vi "statistical test.vi"() -> ()   [LabVIEW 2020]
uses:
  cbe3630c-a9ac-4615-a769-21536e683349.vi
  c04601fd-c9b4-47d5-8825-3c995806f4c0.vi
  2572ad4a-3046-4405-892d-2e3ff8b2e1b5.vi
  <vilib>/Analysis/2dsp.llb/Real FFT.vi
  e90844b8-1ebf-47aa-9ece-e238ecb31719.vi
  c1b2c77b-ae4a-4a6f-8510-2936ba5ac98e.vi
  64edd431-45f5-4cf3-b232-8b968e9fa659.vi
  ced42c1c-8a2c-4fd2-8d95-4dc111501514.vi
  3b9e0fed-1065-4ad9-a1c5-79d92d83ef64.vi
  <vilib>/Utility/file.llb/Read Delimited Spreadsheet (string).vi
  <vilib>/gmath/statdist.llb/Normal CDF.vi
  <vilib>/Comparison/Equal/Equal Functor/Equal Functor.lvclass
  <vilib>/express/express arith-compare/Formula/XNode/ExpressFormulaBlockNode.xnode
  <vilib>/gmath/NI_Gmath.lvlib
  <vilib>/Analysis/NI_AALPro.lvlib
panel:
  out "size(s)":i32
  in  "?":T1(tab)
  out "?":dbl
  out "?":dbl format="%.6f"
  out "?":dbl format="%.6f"
  out "?":dbl format="%.6f"
  out "?":dbl
  out "1 - erf(x)":dbl format="%.6f"
  out "1 - g(x, a)":dbl format="%.6f"
  out "P-VALUE 2":dbl format="%.6f"
  out "p-value 4":dbl format="%.6f"
  out "?":dbl format="%.6f"
  out "?":dbl format="%.6f"
  out "?":dbl format="%.6f"
  out "?":dbl
  out "?":dbl
  out "?":dbl
  out "?":string
  out "?":string
  out "?":string
  out "?":string
  out "?":string
  out "?":string
  out "?":string
  out "?":string
  out "?":string
  out "?":string
  out "?":string
  out "?":string
  out "?":string
  out "?":string
  out "?":string
  out "lxl":i32
  out "Z-":i32
  out "s":dbl
  out "sqrt(Z-)":dbl
  out "s/sqrt(2)":dbl
  out "X":dbl format="%#_8g"
  out "X/2":dbl format="%#_8g"
  out "n/2":dbl
  in  "M 길이":i32
  out "pi":dbl
  out "V(obs)":i32
  out "erfc(  )":dbl
  in  "MAX RUN":i32
  out "X^2":dbl
  out "Array":i32[](array[numeric])
  out "N":dbl
  out "32":dbl
  out "31":dbl
  out "0":dbl
  out "X^2 2":dbl format="%#_8g"
  out "결과":dbl
  in  "차원 크기":i32
  out "log(x)":dbl
  out "T":dbl
  out "N0":dbl format="%#_8g"
  out "N1":dbl format="%#_8g"
  out "x":dbl
  out "d":dbl
  out "u":dbl
  out "시그마^2":dbl
  out "X^2 3":dbl
  out "길이 M":i32
  out "람다":dbl
  out "에타":dbl
  out "v4":i32
  out "v1":i32
  out "v0":i32
  out "v5":i32
  out "v2":i32
  out "v3":i32
  out "X^2 4":dbl format="%#_7g"
  out "f(n)":dbl
  out "c":dbl
  out "시그마":dbl
  out "erfc( )":dbl
  in  "dimension size":i32
  out "v0 2":i32
  out "v1 2":i32
  out "v2 2":i32
  out "v3 2":i32
  out "v4 2":i32
  out "v5 2":i32
  out "v6":i32
  out "전체":i32
  out "안에":i32
  in  "m":i32
  out "델타 프사이":dbl
  out "델타^2 프사이":dbl
  out "2^(m-2)":dbl
  out "2^(m-3)":dbl
  out "p-value2":dbl format="%.6f"
  in  "m 2":i32
  out "ApEn(m)":dbl
  out "X^2 5":dbl format="%#_7g"
  out "forward max value":i32
  out "backward max value":i32
  out "backward P-value":dbl
  out "Forward P-value":dbl
  out "J":i32
  out "P- VALUE":dbl[](array[numeric])
  out "X^2 6":dbl[](array[numeric])
  out "J":i32
  out "P-VALUE":dbl[](array[numeric])
  out "Numeric 3":i32 format="%b"
  out "Numeric 2":i32 format="%b"
  # "Statistical Test                 P-value              Result"
  # "Frequency"
  # "Block Frequency"
  # "Runs"
  # "Long Runs of Ones"
  # "Rank"
  # "FFT"
  # "NON-overlapping Templates"
  # "Overlapping Templates"
  # "Universal"
  # "Linear Complexity"
  # "Serial"
  # "Approximate Entropy"
  # "Cumulative  sum"
  # "Random Excursious"
  # "Random Excursious Variant"
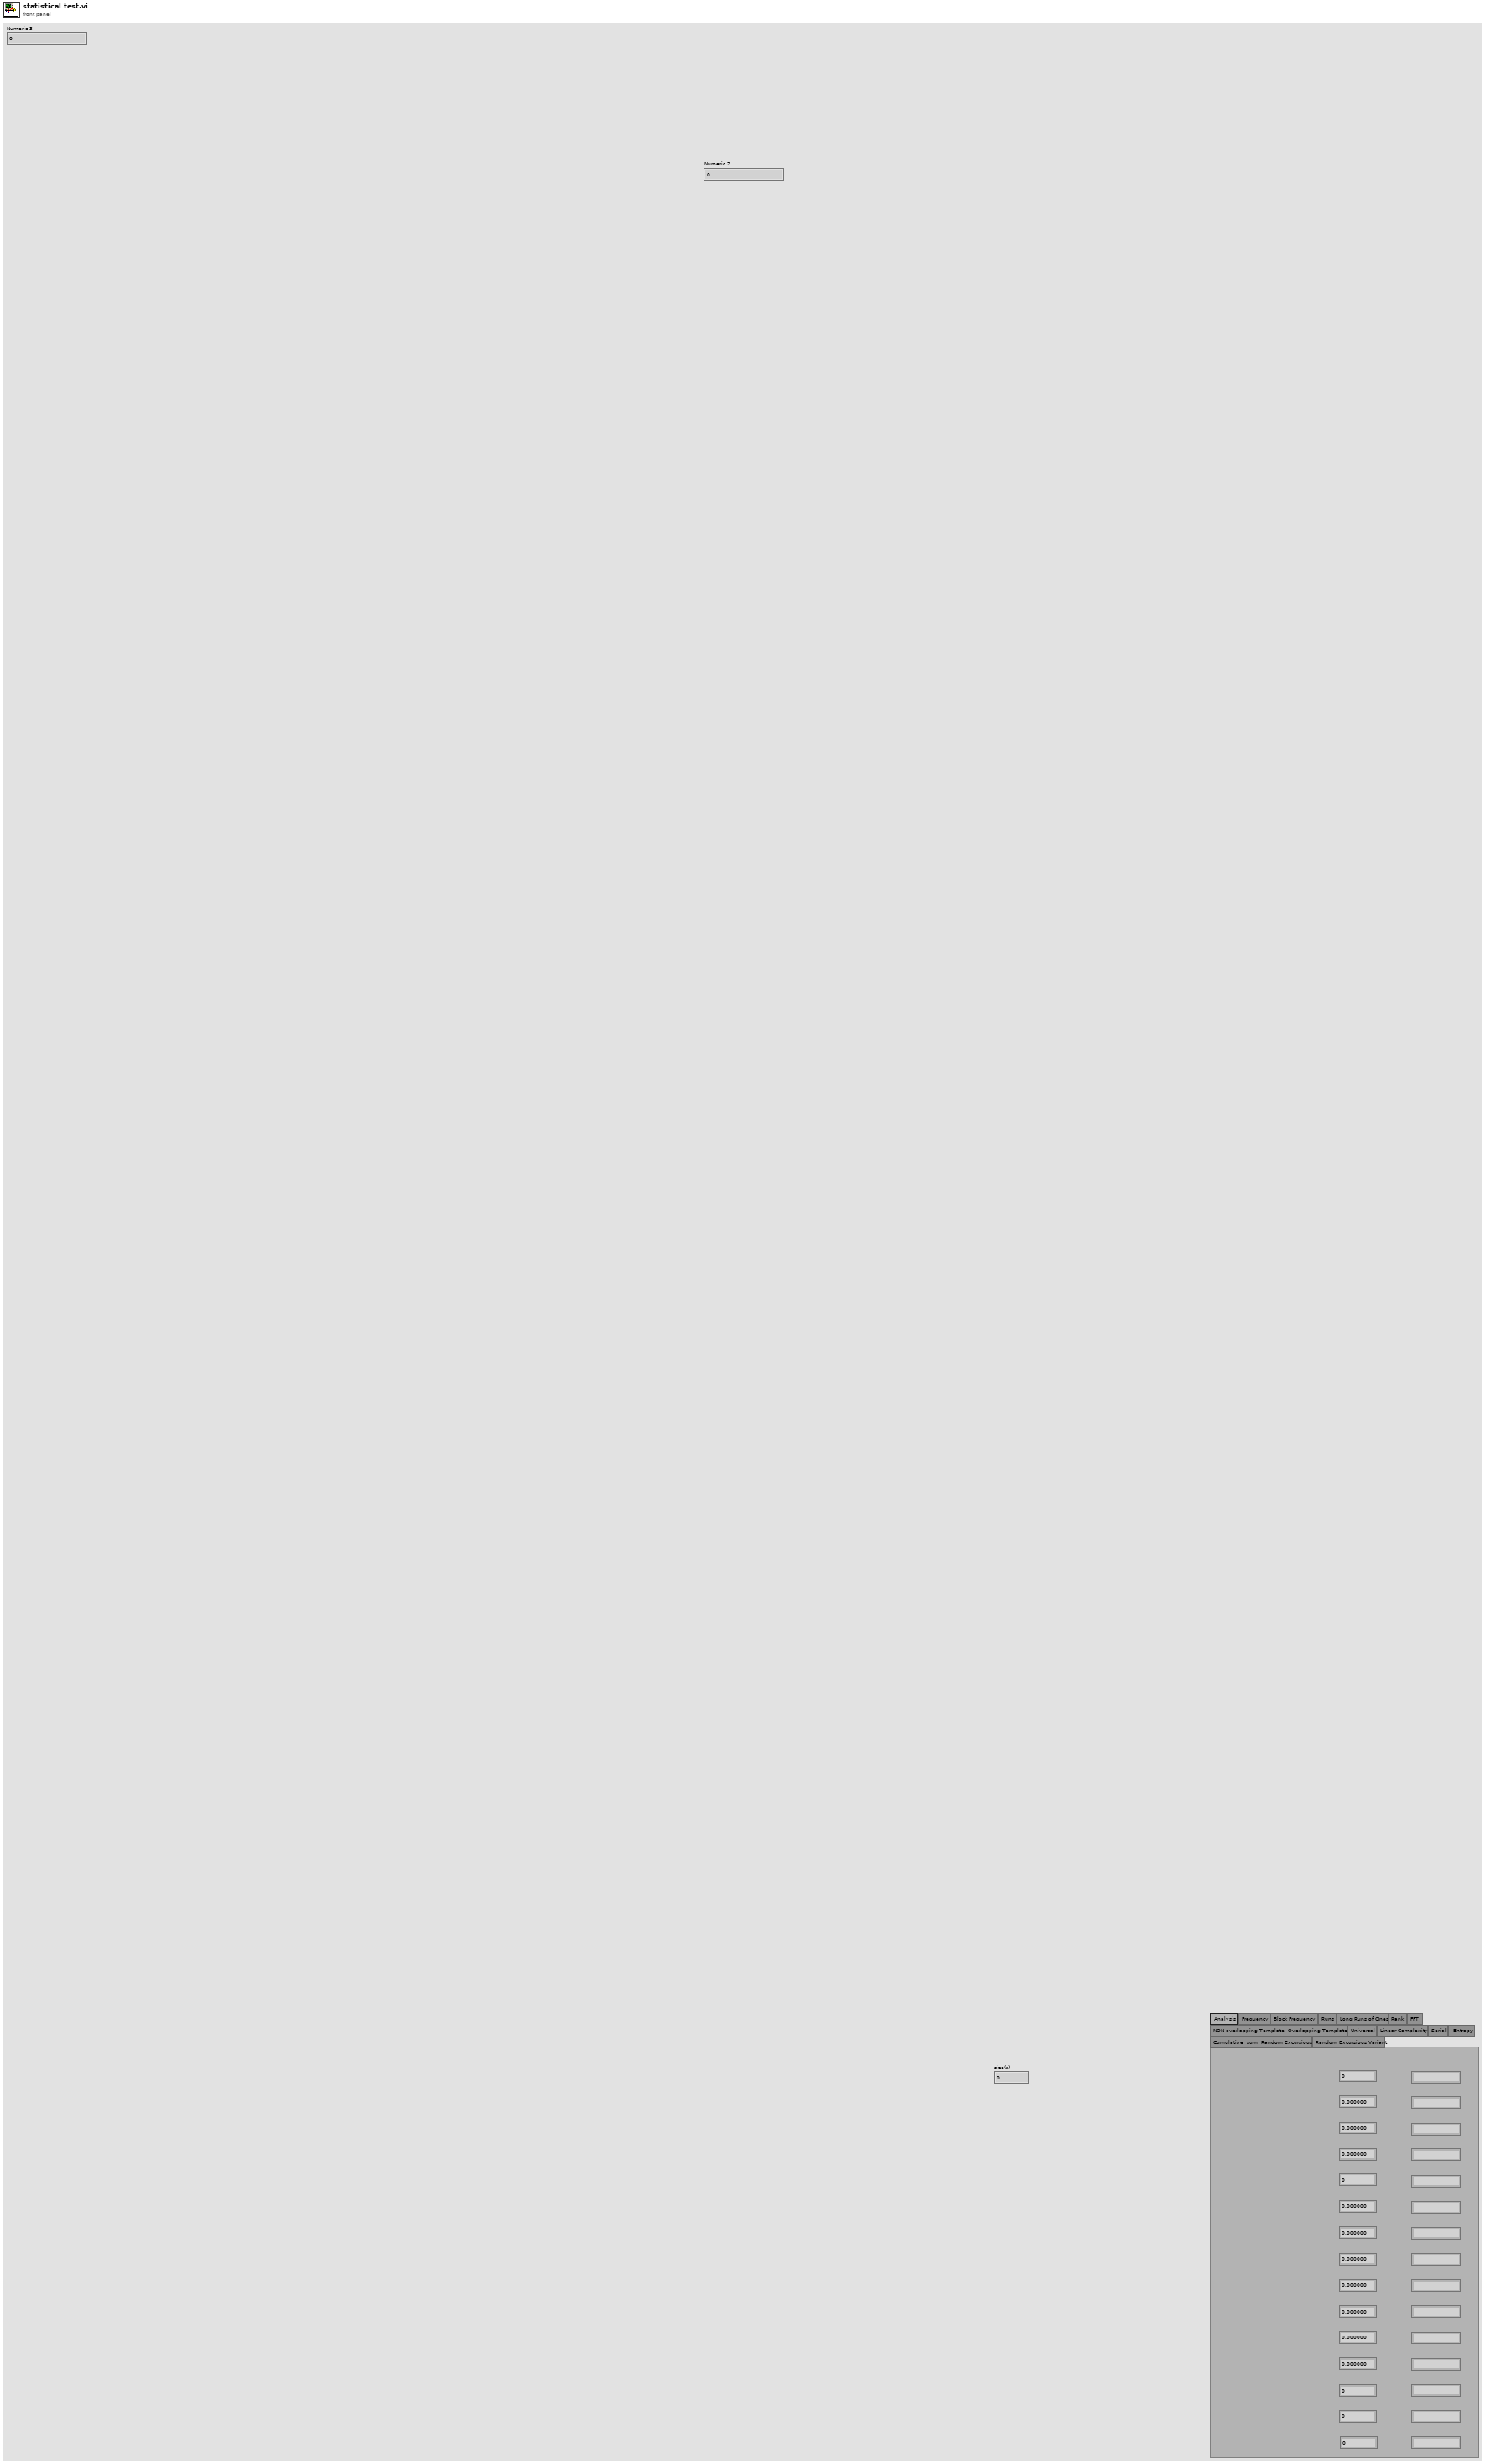
[diagram p1: front panel]
types:
  T1 = enum32{"Analysis ", "Frequency", "Block Frequency", "Runs", "Long Runs of Ones", "Rank", "FFT", "NON-overlapping Templates", "Overlapping Templates", "Universal", "Linear Complexity", "Serial", " Entropy", "Cumulative  sum", "Random Excursious", "Random Excursious Variant"}
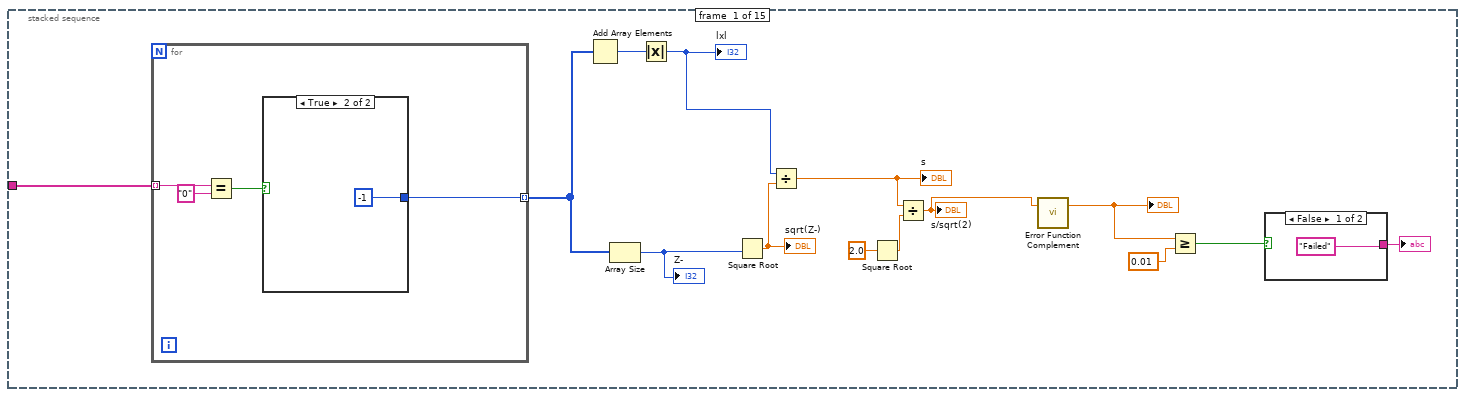
[diagram p2: hidden frame]
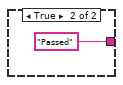
[diagram p3: hidden frame]
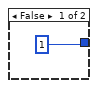
[diagram p4: hidden frame]
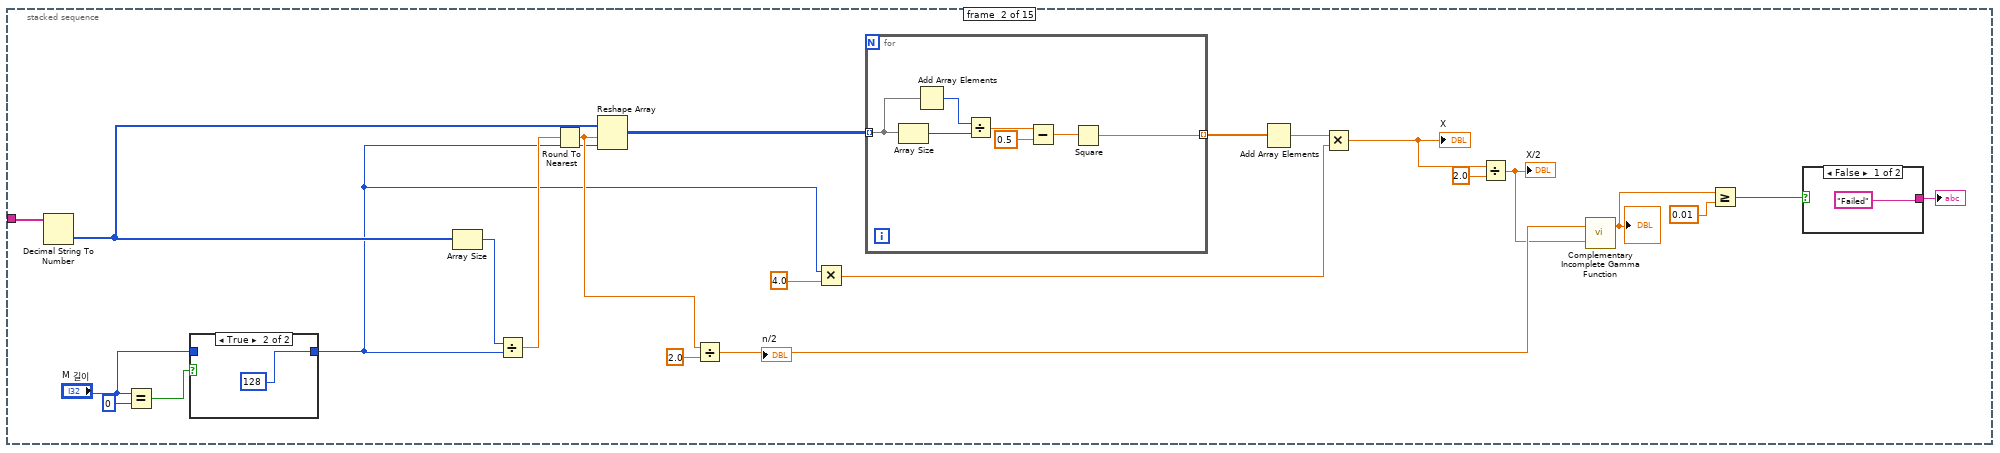
[diagram p5: hidden frame]
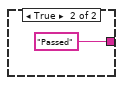
[diagram p7: hidden frame]
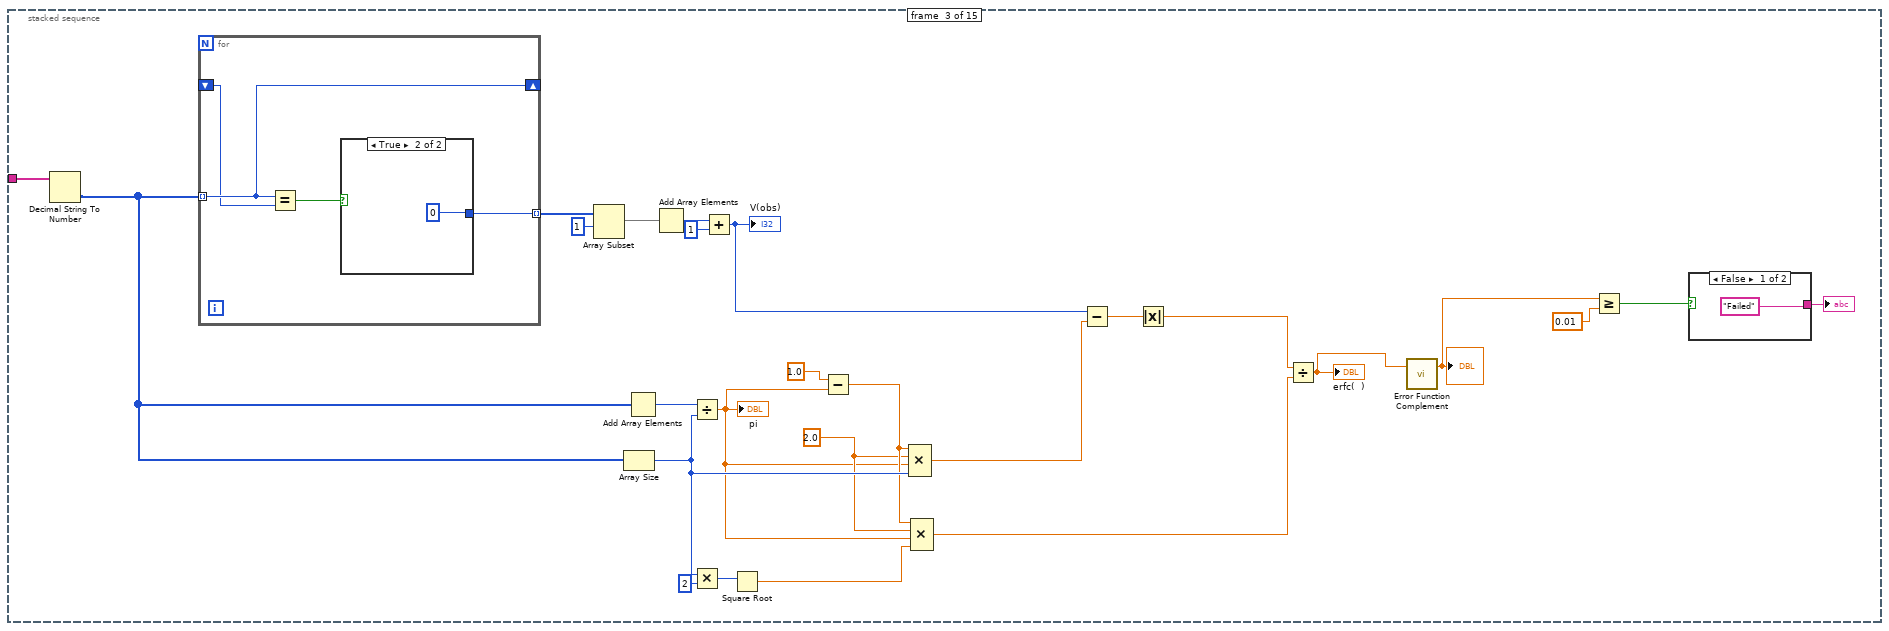
[diagram p8: hidden frame]
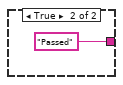
[diagram p9: hidden frame]
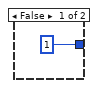
[diagram p10: hidden frame]
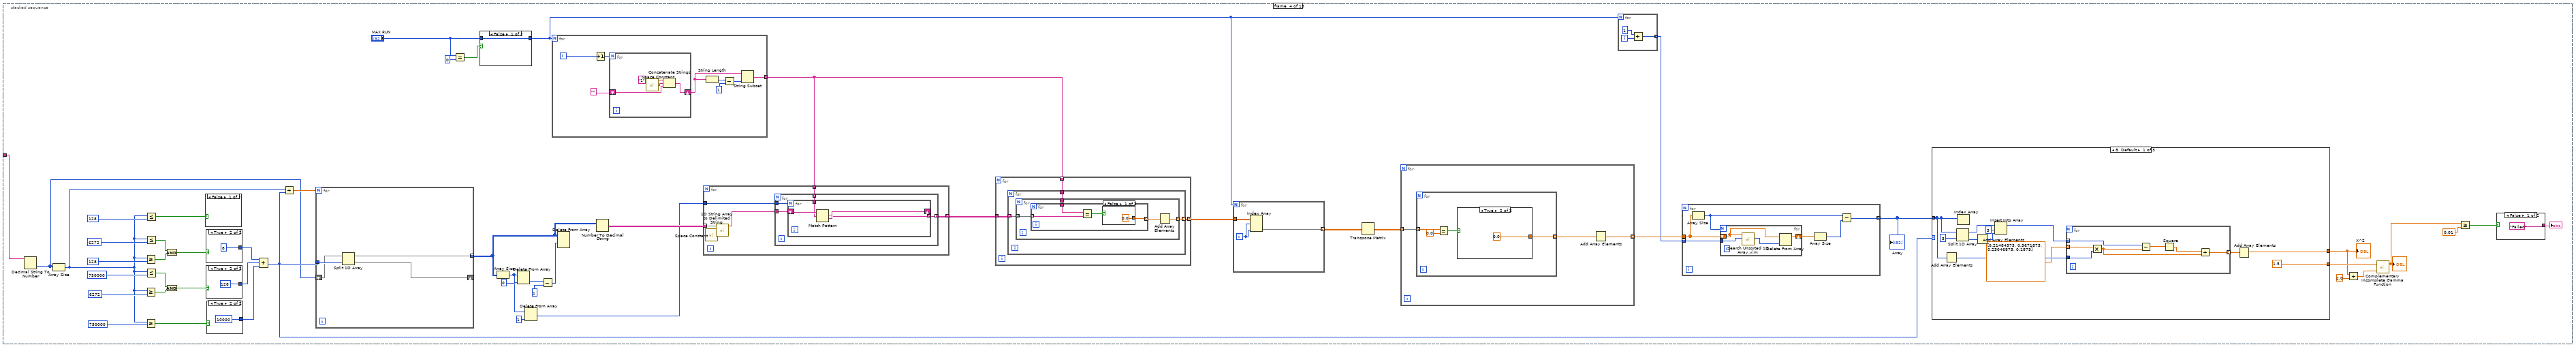
[diagram p11: hidden frame]
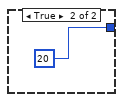
[diagram p12: hidden frame]
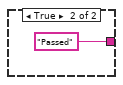
[diagram p13: hidden frame]
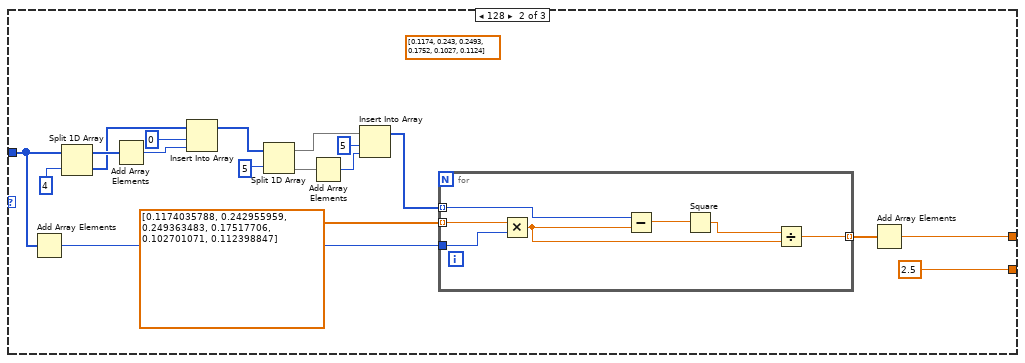
[diagram p14: hidden frame]
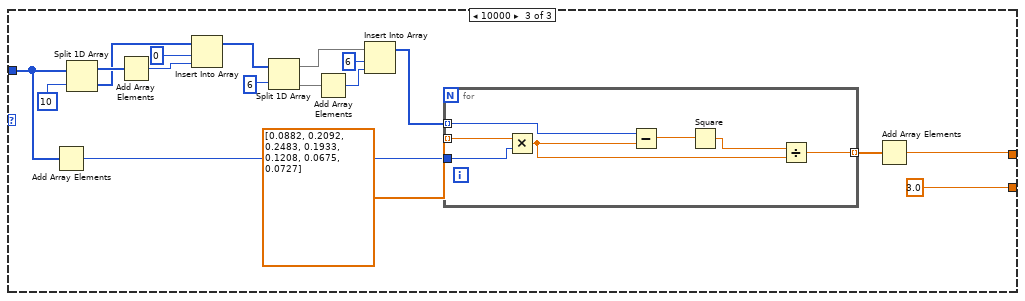
[diagram p15: hidden frame]
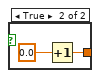
[diagram p16: hidden frame]
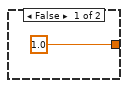
[diagram p17: hidden frame]
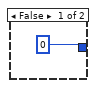
[diagram p19: hidden frame]
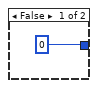
[diagram p20: hidden frame]
diagram:
  n1 = call-poly <vilib>:"Read Delimited Spreadsheet.vi"("file path (dialog if empty)"=path "C:/POST PROCESSING/2진수green only1-2.txt", "number of rows (all:-1)"=-1, "start of read offset (chars.:0)"=0, "max characters/row  (no limit:0)"=0) -> ("first row"=w5:string[])  [unwired: 6 in, 5 out]
  n2 = Array Size(array=w5) -> (size(s)=w14:i32)
  n3 = for {
    N: w14 -> [_]
    tunnel: w5 -> [w17] mode=indexing
    tunnel: [w16] -> w13 mode=indexing
    n4 = String Subset(string=w17, length (rest)=1 ("길이(나머지)")) -> (substring=w16:string)  [unwired: 1 in]
  }
  n5 = for {
    N: w14 -> [_]
    tunnel: w5 -> [w21] mode=indexing
    tunnel: [w20] -> w12 mode=indexing
    n6 = String Subset(string=w21, offset (0)=1 ("오프셋(0)"), length (rest)=1 ("길이(나머지)")) -> (substring=w20:string)
  }
  n7 = for {
    N: w14 -> [_]
    tunnel: w5 -> [w25] mode=indexing
    tunnel: [w24] -> w10 mode=indexing
    n8 = String Subset(string=w25, offset (0)=3 ("오프셋(0)"), length (rest)=1 ("길이(나머지)")) -> (substring=w24:string)
  }
  n9 = for {
    N: w14 -> [_]
    tunnel: w5 -> [w29] mode=indexing
    tunnel: [w28] -> w11 mode=indexing
    n10 = String Subset(string=w29, offset (0)=2 ("오프셋(0)"), length (rest)=1 ("길이(나머지)")) -> (substring=w28:string)
  }
  n11 = Interleave 1D Arrays(w13, w12, w11, w10) -> (w4:string[])
  n12 = Reshape Array(w4, 6400000 ("dimension size")) -> (w2:string[])
  n13 = Array Size(array=w2) -> (size(s)=→"size(s)":i32)
  n14 = stacked-sequence {
    tunnel: w2 -> [w34 w60 w90 w128 w327 w692 w739 w807 w983 w1233 w1509 w1620 w1729 w1863 w1994]
    frame #0 {
      n15 = for {
        tunnel: w34 -> [w49] mode=indexing
        tunnel: [w46] -> w42 mode=indexing
        n16 = Equal?(x=w49, y="0") -> (x = y?=w47:bool)
        n17 = case shown="True" w47 {
          tunnel: [1 -1] -> w46
          frame False {
          }
          frame True {
          }
        }
      }
      n18 = Add Array Elements(numeric array=w42) -> (sum=w43:i32)
      n19 = Array Size(array=w42) -> (size(s)=w40:i32)
      "Z-" <- w40
      n20 = Absolute Value(x=w43) -> (abs(x)=w41:i32)
      "lxl" <- w41
      n21 = Square Root(x=w40) -> (sqrt(x)=w39:dbl)
      "sqrt(Z-)" <- w39
      n22 = Divide(x=w41, y=w39) -> (x/y=w36:dbl)
      "s" <- w36
      n23 = Square Root(x=2.0) -> (sqrt(x)=w37:dbl)
      n24 = Divide(x=w36, y=w37) -> (x/y=w35:dbl)
      "s/sqrt(2)" <- w35
      n25 = call <vilib>:"Error Function Complement.vi"("x"=w35) -> ("1 - erf(x)"=w30:dbl)  [unwired: 2 in]
      "?" <- w30
      n26 = Greater Or Equal?(x=w30, y=0.01) -> (x >= y?=w32:bool)
      n27 = case shown="False" w32 {
        tunnel: ["Failed" "Passed"] -> w31
        frame False {
        }
        frame True {
        }
      }
      "?" <- w31
    }
    frame #1 {
      n28 = Decimal String To Number(string=w60) -> (number=w66:i32[])  [unwired: 2 in, 1 out]
      n29 = Equal?(x="M 길이", y=0) -> (x = y?=w54:bool)
      n30 = case shown="True" w54 {
        tunnel: [w75 128] -> w52
        tunnel: "M 길이" -> [w75 _]
        frame False {
        }
        frame True {
        }
      }
      n31 = Array Size(array=w66) -> (size(s)=w64:i32)
      n32 = Divide(x=w64, y=w52) -> (x/y=w62:dbl)
      n33 = Round To Nearest(number=w62) -> (nearest integer value=w61:dbl)
      n34 = Reshape Array(w66, w61, w52) -> (w65:i32[][])
      n35 = Divide(x=w61, y=2.0) -> (x/y=w68:dbl)
      "n/2" <- w68
      n36 = Multiply(x=w52, y=4.0) -> (x*y=w72:dbl)
      n37 = for {
        tunnel: w65 -> [w85] mode=indexing
        tunnel: [w80] -> w74 mode=indexing
        n38 = Array Size(array=w85) -> (size(s)=w79:i32)
        n39 = Add Array Elements(numeric array=w85) -> (sum=w84:i32)
        n40 = Divide(x=w84, y=w79) -> (x/y=w83:dbl)
        n41 = Subtract(x=w83, y=0.5) -> (x-y=w81:dbl)
        n42 = Square(x=w81) -> (x^2=w80:dbl)
      }
      n43 = Add Array Elements(numeric array=w74) -> (sum=w73:dbl)
      n44 = Multiply(x=w73, y=w72) -> (x*y=w71:dbl)
      "X" <- w71
      n45 = Divide(x=w71, y=2.0) -> (x/y=w67:dbl)
      "X/2" <- w67
      n46 = call <vilib>:"Complementary Incomplete Gamma Function.vi"("a"=w67, "x"=w68) -> ("1 - g(x, a)"=w56:dbl)  [unwired: 1 in]
      "?" <- w56
      n47 = Greater Or Equal?(x=w56, y=0.01) -> (x >= y?=w58:bool)
      n48 = case shown="False" w58 {
        tunnel: ["Failed" "Passed"] -> w57
        frame False {
        }
        frame True {
        }
      }
      "?" <- w57
    }
    frame #2 {
      w97 = 2.0 ("x")
      n49 = Decimal String To Number(string=w90) -> (number=w91:i32[])  [unwired: 2 in, 1 out]
      n50 = for {
        tunnel: w91 -> [w117] mode=indexing
        shift-right: [w117] -> _
        shift-left: _ -> [w116]
        tunnel: [w114] -> w109 mode=indexing
        n51 = Equal?(x=w117, y=w116) -> (x = y?=w115:bool)
        n52 = case shown="True" w115 {
          tunnel: [1 0] -> w114
          frame False {
          }
          frame True {
          }
        }
      }
      n53 = Array Subset(array=w109, index=1 ("인덱스")) -> (w108:i32[])  [unwired: 1 in]
      n54 = Array Size(array=w91) -> (size(s)=w101:i32)
      n55 = Add Array Elements(numeric array=w91) -> (sum=w111:i32)
      n56 = Add Array Elements(numeric array=w108) -> (sum=w107:i32)
      n57 = Divide(x=w111, y=w101) -> (x/y=w96:dbl)
      "pi" <- w96
      n58 = Multiply(x=w101, y=2) -> (x*y=w99:i32)
      n59 = Add(x=w107, y=1) -> (x+y=w104:i32)
      "V(obs)" <- w104
      n60 = Square Root(x=w99) -> (sqrt(x)=w95:dbl)
      n61 = Subtract(x=1.0, y=w96) -> (x-y=w98:dbl)
      n62 = Compound Arithmetic op=MULTIPLY(w98, w97, w96, w101) -> (w103:dbl)
      n63 = Compound Arithmetic op=MULTIPLY(w98, w97, w96, w95) -> (w93:dbl)
      n64 = Subtract(x=w104, y=w103) -> (x-y=w102:dbl)
      n65 = Absolute Value(x=w102) -> (abs(x)=w94:dbl)
      n66 = Divide(x=w94, y=w93) -> (x/y=w92:dbl)
      "erfc(  )" <- w92
      n67 = call <vilib>:"Error Function Complement.vi"("x"=w92) -> ("1 - erf(x)"=w86:dbl)  [unwired: 2 in]
      "?" <- w86
      n68 = Greater Or Equal?(x=w86, y=0.01) -> (x >= y?=w88:bool)
      n69 = case shown="False" w88 {
        tunnel: ["Failed" "Passed"] -> w87
        frame False {
        }
        frame True {
        }
      }
      "?" <- w87
    }
    frame #3 {
      n70 = Decimal String To Number(string=w128) -> (number=w129:i32[])  [unwired: 2 in, 1 out]
      n71 = Array Size(array=w129) -> (size(s)=w155:i32)
      n72 = Greater Or Equal?(x=w155, y=128) -> (x >= y?=w161:bool)
      n73 = Greater Or Equal?(x=w155, y=6272) -> (x >= y?=w163:bool)
      n74 = Greater Or Equal?(x=w155, y=750000) -> (x >= y?=w158:bool)
      n75 = Less Or Equal?(x=w155, y=128) -> (x <= y?=w157:bool)
      n76 = Less Or Equal?(x=w155, y=6272) -> (x <= y?=w162:bool)
      n77 = Less Or Equal?(x=w155, y=750000) -> (x <= y?=w164:bool)
      n78 = And(x=w162, y=w161) -> (x .and. y?=w160:bool)
      n79 = And(x=w164, y=w163) -> (x .and. y?=w159:bool)
      n80 = case shown="False" w157 {
        frame False {
        }
        frame True {
        }
      }
      n81 = case shown="True" w160 {
        tunnel: [0 8] -> w156
        frame False {
        }
        frame True {
        }
      }
      n82 = case shown="True" w159 {
        tunnel: [0 128] -> w147
        frame False {
        }
        frame True {
        }
      }
      n83 = case shown="True" w158 {
        tunnel: [0 10000] -> w146
        frame False {
        }
        frame True {
        }
      }
      n84 = Compound Arithmetic op=ADD(w156, w147, w146) -> (w135:i32)
      n85 = Divide(x=w155, y=w135) -> (x/y=w154:dbl)
      n86 = for {
        N: w154 -> [_]
        tunnel: w135 -> [w321]
        shift-right: [w319] -> _
        shift-left: w129 -> [w320]
        tunnel: [w318] -> w145 mode=indexing
        n87 = Split 1D Array(array=w320, index=w321) -> (first subarray=w318:i32[], second subarray=w319:i32[])
      }
      n88 = Equal?(x="MAX RUN", y=0) -> (x = y?=w122:bool)
      n89 = case shown="False" w122 {
        tunnel: [w171 20] -> w120
        tunnel: "MAX RUN" -> [w171 _]
        frame False {
        }
        frame True {
        }
      }
      n90 = Array Size(array=w145) -> (size(s)=w148:i32[])
      n91 = Delete From Array(array=w148, index=0 ("인덱스")) -> (deleted portion=w151:i32)  [unwired: 1 in, 1 out]
      n92 = Delete From Array(array=w148, index=1 ("인덱스")) -> (deleted portion=w143:i32)  [unwired: 1 in, 1 out]
      n93 = Subtract(x=w151, y=1) -> (x-y=w152:i32)
      n94 = for {
        N: w120 -> [_]
        tunnel: [w279] -> w140 mode=indexing
        i -> [w278]
        n95 = Increment(x=w278) -> (x+1=w277:i32)
        n96 = for {
          N: w277 -> [_]
          shift-right: [w287] -> w282
          shift-left: "" -> [w285]
          n97 = call <vilib>:"Space Constant.vi"() -> ("String"=w286:string)
          n98 = Concatenate Strings("1" ("string"), w286, w285) -> (w287:string)
        }
        n99 = String Length(string=w282) -> (length=w283:i32)
        n100 = Subtract(x=w283, y=1) -> (x-y=w284:i32)
        n101 = String Subset(string=w282, length (rest)=w284) -> (substring=w279:string)  [unwired: 1 in]
      }
      n102 = Delete From Array(array=w145, index (row)=w152) -> ()  [unwired: 2 in, 2 out]
      n103 = Number To Decimal String(number=w145) -> (decimal integer string=w144:string[][])  [unwired: 1 in]
      n104 = for {
        tunnel: w144 -> [w294] mode=indexing
        tunnel: [w292] -> w142 mode=indexing
        tunnel: w143 -> [w291]
        tunnel: w140 -> [w289]
        n105 = call <vilib>:"Space Constant.vi"() -> ("String"=w290:string)
        n106 = call <vilib>:"1D String Array to Delimited String.vi"("delimiter"=w290, "string array"=w294) -> ("delimited string"=w293:string)  [unwired: 9 in]
        n107 = for {
          tunnel: w293 -> [w298]
          tunnel: [w297] -> w292 mode=indexing
          tunnel: w291 -> [w296]
          tunnel: w289 -> [w295] mode=indexing
          n108 = for {
            N: w296 -> [_]
            shift-right: [w301] -> _
            shift-left: w298 -> [w302]
            tunnel: [w300] -> w297 mode=indexing
            tunnel: w295 -> [w299]
            n109 = Match Pattern(string=w302, regular expression=w299) -> (match substring=w300:string, after substring=w301:string)  [unwired: 1 in, 2 out]
          }
        }
      }
      n110 = for {
        tunnel: w142 -> [w262]
        tunnel: [w261] -> w141 mode=indexing
        tunnel: w140 -> [w260] mode=indexing
        n111 = for {
          tunnel: w262 -> [w265] mode=indexing
          tunnel: [w264] -> w261 mode=indexing
          tunnel: w260 -> [w263]
          n112 = for {
            tunnel: w265 -> [w269] mode=indexing
            tunnel: [w267] -> w264 mode=indexing
            tunnel: w263 -> [w266]
            n113 = for {
              tunnel: w269 -> [w271] mode=indexing
              tunnel: [w272] -> w268 mode=indexing
              tunnel: w266 -> [w270]
              n114 = Equal?(x=w270, y=w271) -> (x = y?=w273:bool)
              n115 = case shown="False" w273 {
                tunnel: [0.0 w275] -> w272
                frame False {
                }
                frame True {
                  n116 = Increment(x=0.0) -> (x+1=w275:dbl)
                }
              }
            }
            n117 = Add Array Elements(numeric array=w268) -> (sum=w267:dbl)
          }
        }
      }
      n118 = for {
        N: w120 -> [_]
        tunnel: w141 -> [w259]
        tunnel: [w257] -> w139 mode=indexing
        i -> [w258]
        n119 = Index Array(array=w259, index (dim 0)=w258, index (dim 2)=w258) -> (element=w257:dbl[])  [unwired: 1 in]
      }
      n120 = Transpose Matrix(1:w139) -> (0:w138:dbl[][])
      n121 = for {
        tunnel: w138 -> [w305] mode=indexing
        tunnel: [w303] -> w136 mode=indexing
        n122 = for {
          tunnel: w305 -> [w309] mode=indexing
          tunnel: [w306] -> w304 mode=indexing
          n123 = Equal?(x=w309, y=0.0) -> (x = y?=w307:bool)
          n124 = case shown="True" w307 {
            tunnel: [1.0 ("y") 0.0 ("y")] -> w306
            frame False {
            }
            frame True {
            }
          }
        }
        n125 = Add Array Elements(numeric array=w304) -> (sum=w303:dbl)
      }
      n126 = for {
        N: w120 -> [_]
        tunnel: [w244] -> w137 mode=indexing
        i -> [w246]
        n127 = Add(x=1, y=w246) -> (x+y=w244:i32)
      }
      n128 = for {
        tunnel: w136 -> [w247]
        tunnel: [w250] -> w131 mode=indexing
        tunnel: w137 -> [w248] mode=indexing
        n129 = Array Size(array=w247) -> (size(s)=w249:i32)
        n130 = for {
          N: w249 -> [_]
          shift-right: [w254] -> w251
          shift-left: w247 -> [w256]
          tunnel: w248 -> [w253]
          n131 = call "Search Unsorted 1D Array.vim"("element"=w253, "unsorted 1D array"=w256) -> ("index of element"=w255:i32)  [unwired: 9 in]
          n132 = Delete From Array(array=w256, index=w255) -> (array with subset deleted=w254:dbl[])  [unwired: 1 in, 1 out]
        }
        n133 = Array Size(array=w251) -> (size(s)=w252:i32)
        n134 = Subtract(x=w249, y=w252) -> (x-y=w250:i32)
      }
      "Array" <- w131
      n135 = case shown="8, Default" w135 {
        tunnel: [w177 w197 w222] -> w130
        tunnel: [1.5 ("x") 2.5 ("x") 3.0 ("x")] -> w132
        tunnel: w131 -> [w176 w196 w220]
        frame 8, Default {
          n136 = Add Array Elements(numeric array=w176) -> (sum=w175:i32)
          n137 = Split 1D Array(array=w176, index=3) -> (first subarray=w183:i32[], second subarray=w184:i32[])
          n138 = Index Array(array=w176) -> ()  [unwired: 1 in, 1 out]
          n139 = Add Array Elements(numeric array=w184) -> (sum=w180:i32)
          n140 = Insert Into Array(array=w183, index=3, new element=w180) -> (w179:i32[])
          n141 = for {
            tunnel: dbl[] [0.21484375, 0.3671875, 0.23046875, 0.1875] -> [w190] mode=indexing
            tunnel: w179 -> [w189] mode=indexing
            tunnel: [w188] -> w178 mode=indexing
            tunnel: w175 -> [w187]
            n142 = Multiply(x=w190, y=w187) -> (x*y=w193:dbl)
            n143 = Subtract(x=w189, y=w193) -> (x-y=w192:dbl)
            n144 = Square(x=w192) -> (x^2=w191:dbl)
            n145 = Divide(x=w191, y=w193) -> (x/y=w188:dbl)
          }
          n146 = Add Array Elements(numeric array=w178) -> (sum=w177:dbl)
        }
        frame 128 {
          (unwired) dbl[] [0.1174, 0.243, 0.2493, 0.1752, 0.1027, 0.1124]
          n147 = Add Array Elements(numeric array=w196) -> (sum=w195:i32)
          n148 = Split 1D Array(array=w196, index=4) -> (first subarray=w208:i32[], second subarray=w207:i32[])
          n149 = Add Array Elements(numeric array=w208) -> (sum=w206:i32)
          n150 = Insert Into Array(array=w207, index=0, new element=w206) -> (w199:i32[])
          n151 = Split 1D Array(array=w199, index=5) -> (first subarray=w203:i32[], second subarray=w204:i32[])
          n152 = Add Array Elements(numeric array=w204) -> (sum=w200:i32)
          n153 = Insert Into Array(array=w203, index=5, new element=w200) -> (w198:i32[])
          n154 = for {
            tunnel: dbl[] [0.1174035788, 0.242955959, 0.249363483, 0.17517706, 0.102701071, 0.112398847] -> [w215] mode=indexing
            tunnel: w198 -> [w214] mode=indexing
            tunnel: [w213] -> w209 mode=indexing
            tunnel: w195 -> [w212]
            n155 = Multiply(x=w215, y=w212) -> (x*y=w218:dbl)
            n156 = Subtract(x=w214, y=w218) -> (x-y=w217:dbl)
            n157 = Square(x=w217) -> (x^2=w216:dbl)
            n158 = Divide(x=w216, y=w218) -> (x/y=w213:dbl)
          }
          n159 = Add Array Elements(numeric array=w209) -> (sum=w197:dbl)
        }
        frame 10000 {
          n160 = Add Array Elements(numeric array=w220) -> (sum=w219:i32)
          n161 = Split 1D Array(array=w220, index=10) -> (first subarray=w234:i32[], second subarray=w233:i32[])
          n162 = Add Array Elements(numeric array=w234) -> (sum=w232:i32)
          n163 = Insert Into Array(array=w233, index=0, new element=w232) -> (w225:i32[])
          n164 = Split 1D Array(array=w225, index=6) -> (first subarray=w229:i32[], second subarray=w230:i32[])
          n165 = Add Array Elements(numeric array=w230) -> (sum=w226:i32)
          n166 = Insert Into Array(array=w229, index=6, new element=w226) -> (w224:i32[])
          n167 = for {
            tunnel: dbl[] [0.0882, 0.2092, 0.2483, 0.1933, 0.1208, 0.0675, 0.0727] -> [w240] mode=indexing
            tunnel: w224 -> [w239] mode=indexing
            tunnel: [w238] -> w235 mode=indexing
            tunnel: w219 -> [w237]
            n168 = Multiply(x=w240, y=w237) -> (x*y=w243:dbl)
            n169 = Subtract(x=w239, y=w243) -> (x-y=w242:dbl)
            n170 = Square(x=w242) -> (x^2=w241:dbl)
            n171 = Divide(x=w241, y=w243) -> (x/y=w238:dbl)
          }
          n172 = Add Array Elements(numeric array=w235) -> (sum=w222:dbl)
        }
      }
      "X^2" <- w130
      n173 = Divide(x=w130, y=2.0) -> (x/y=w134:dbl)
      n174 = call <vilib>:"Complementary Incomplete Gamma Function.vi"("a"=w134, "x"=w132) -> ("1 - g(x, a)"=w124:dbl)  [unwired: 1 in]
      "?" <- w124
      n175 = Greater Or Equal?(x=w124, y=0.01) -> (x >= y?=w126:bool)
      n176 = case shown="False" w126 {
        tunnel: ["Failed" "Passed"] -> w125
        frame False {
        }
        frame True {
        }
      }
      "?" <- w125
    }
    frame #4 {
      (unwired) 1.0 ("y")
      n177 = Decimal String To Number(string=w327) -> (number=w342:i32[])  [unwired: 2 in, 1 out]
      n178 = Array Size(array=w342) -> (size(s)=w366:i32)
      n179 = Divide(x=w366, y=32) -> (x/y=w336:dbl)
      n180 = Round Toward -Infinity(1:w336) -> (0:w335:dbl)
      n181 = for {
        N: w335 -> [_]
        shift-right: [w685] -> _
        shift-left: w342 -> [w686]
        tunnel: [w684] -> w363 mode=indexing
        n182 = Split 1D Array(array=w686, index=32 ("인덱스")) -> (first subarray=w684:i32[], second subarray=w685:i32[])
      }
      n183 = Divide(x=w335, y=32) -> (x/y=w322:dbl)
      n184 = Reshape Array(w342, w322, "차원 크기", "차원 크기") -> ()  [unwired: 1 out]
      n185 = Round To Nearest(number=w322) -> (nearest integer value=w331:dbl)
      "N" <- w331
      n186 = for {
        N: w322 -> [_]
        tunnel: w363 -> [w683]
        tunnel: [w672] -> w341 mode=indexing
        i -> [w676]
        n187 = Add(x=1, y=w676) -> (x+y=w680:i32)
        n188 = Multiply(x=32.0, y=w676) -> (x*y=w675:dbl)
        n189 = Multiply(x=32.0, y=w680) -> (x*y=w679:dbl)
        n190 = Subtract(x=w679, y=1.0) -> (x-y=w674:dbl)
        n191 = Array Subset(array=w683, index (row)=w675, length (row)=w674, length (col)=31 ("열 N")) -> (w672:dbl[][])  [unwired: 1 in]
      }
      n192 = for {
        tunnel: w341 -> [w559] mode=indexing
        tunnel: [w558] -> w362 mode=indexing
        n193 = Index Array(array=w559, index (row)=0 ("인덱스 (행)"), index (col)=0 ("인덱스 (열)")) -> (element=w562:dbl[][])
        n194 = Delete From Array(array=w562, index (col)=0 ("비활성화된 인덱스 (열)")) -> (deleted portion=w560:dbl[])  [unwired: 2 in, 1 out]
        n195 = for {
          tunnel: w560 -> [_] mode=indexing
          shift-right: [w575] -> w558
          shift-left: w559 -> [w565]
          i -> [w567]
          # "대각성분이 1일떄"
          n196 = Index Array(array=w565, index (row)=0 ("인덱스 (행)"), index (col)=0 ("인덱스 (열)")) -> (element=w570:dbl[][])
          n197 = Delete From Array(array=w570, index (col)=0 ("비활성화된 인덱스 (열)")) -> (deleted portion=w568:dbl[])  [unwired: 2 in, 1 out]
          n198 = Add(x=w567, y=1) -> (x+y=w574:i32)
          n199 = Delete From Array(array=w565, index (col)=w567) -> (deleted portion=w582:dbl[])  [unwired: 2 in, 1 out]
          n200 = Index Array(array=w568, index=w567) -> (element=w566:dbl)
          n201 = Equal?(x=w566, y=1.0) -> (x = y?=w577:bool)
          n202 = Split 1D Array(array=w582, index=w574) -> (second subarray=w578:dbl[])  [unwired: 1 out]
          n203 = call "Search Unsorted 1D Array.vim"("element"=1.0, "unsorted 1D array"=w578) -> ("index of element"=w580:i32)  [unwired: 9 in]
          n204 = Add(x=1, y=w580) -> (x+y=w573:i32)
          n205 = for {
            N: 1 -> [_]
            tunnel: w577 -> [w593]
            tunnel: w567 -> [w592]
            tunnel: w574 -> [w591]
            tunnel: w578 -> [w590]
            tunnel: w573 -> [w589]
            shift-right: [w588] -> w575
            shift-left: w565 -> [w585]
            tunnel: w567 -> [w587]
            tunnel: w574 -> [w586]
            n206 = case shown="False" w593 {
              tunnel: w590 -> [w602 w652]
              tunnel: w591 -> [w601 w654]
              tunnel: w585 -> [w598 w651]
              tunnel: w592 -> [w600 w653]
              tunnel: [w597 w650] -> w588
              tunnel: w592 -> [w599 _]
              tunnel: w589 -> [w596 _]
              tunnel: w587 -> [w595 _]
              tunnel: w586 -> [w594 _]
              frame False {
                n207 = for {
                  N: w596 -> [_]
                  tunnel: w602 -> [w611] mode=indexing
                  tunnel: w601 -> [w614]
                  tunnel: w600 -> [w612]
                  tunnel: w599 -> [w610]
                  shift-right: [w605] -> w597
                  shift-left: w598 -> [w606]
                  tunnel: w595 -> [w604]
                  tunnel: w594 -> [w603]
                  i -> [w607]
                  # "대각성분으로 넘어가야됨"
                  # "1처음나온거 바꾸고 그만해야됨"
                  n208 = Equal?(x=w611, y=1.0) -> (x = y?=w615:bool)
                  n209 = Add(x=w614, y=w607) -> (x+y=w613:i32)
                  n210 = Add(x=1, y=w607) -> (x+y=w608:i32)
                  n211 = case shown="True" w615 {
                    tunnel: w613 -> [_ w628]
                    tunnel: w612 -> [_ w630]
                    tunnel: w606 -> [w617 w632]
                    tunnel: w610 -> [_ w625]
                    tunnel: w608 -> [_ _]
                    tunnel: w604 -> [_ w619]
                    tunnel: [w617 w620] -> w605
                    tunnel: w603 -> [_ w618]
                    frame False {
                    }
                    frame True {
                      n212 = Delete From Array(array=w632, index (row)=w630) -> (deleted portion=w621:dbl[])  [unwired: 2 in, 1 out]
                      n213 = Delete From Array(array=w632, index (row)=w628) -> (deleted portion=w629:dbl[])  [unwired: 2 in, 1 out]
                      n214 = Replace Array Subset(array=w632, new element=w621, index (row)=w628) -> (w631:dbl[][])  [unwired: 1 in]
                      n215 = Replace Array Subset(array=w631, new element=w629, index (row)=w630) -> (w626:dbl[][])  [unwired: 1 in]
                      n216 = Delete From Array(array=w626, index (col)=w625) -> (deleted portion=w627:dbl[])  [unwired: 2 in, 1 out]
                      n217 = Add(x=w625, y=1) -> (x+y=w623:i32)
                      n218 = Split 1D Array(array=w627, index=w623) -> (second subarray=w622:dbl[])  [unwired: 1 out]
                      n219 = for {
                        tunnel: w622 -> [w635] mode=indexing
                        tunnel: w618 -> [w638]
                        tunnel: w619 -> [w636]
                        shift-right: [w634] -> w620
                        shift-left: w626 -> [w633]
                        i -> [w639]
                        n220 = Equal?(x=w635, y=1.0) -> (x = y?=w640:bool)
                        n221 = Add(x=w638, y=w639) -> (x+y=w637:i32)
                        n222 = case shown="True" w640 {
                          tunnel: w637 -> [_ w645]
                          tunnel: w636 -> [_ w649]
                          tunnel: w633 -> [w642 w646]
                          tunnel: [w642 w643] -> w634
                          frame False {
                          }
                          frame True {
                            # "32번안돌고 442 ,557번돔"
                            n223 = Delete From Array(array=w646, index (row)=w649) -> (deleted portion=w647:dbl[])  [unwired: 2 in, 1 out]
                            n224 = Delete From Array(array=w646, index (row)=w645) -> (deleted portion=w648:dbl[])  [unwired: 2 in, 1 out]
                            n225 = Exclusive Or(1:w648, 2:w647) -> (0:w644:i32[])
                            n226 = Replace Array Subset(array=w646, new element=w644, index (row)=w645) -> (w643:dbl[][])  [unwired: 1 in]
                          }
                        }
                      }
                    }
                  }
                }
              }
              frame True {
                n227 = for {
                  tunnel: w652 -> [w659] mode=indexing
                  tunnel: w654 -> [w662]
                  tunnel: w653 -> [w660]
                  shift-right: [w657] -> w650
                  shift-left: w651 -> [w656]
                  i -> [w663]
                  # "1열에서 1이 있는지"
                  n228 = Equal?(x=w659, y=1.0) -> (x = y?=w658:bool)
                  n229 = Add(x=w662, y=w663) -> (x+y=w661:i32)
                  n230 = case shown="True" w658 {
                    tunnel: w661 -> [_ w666]
                    tunnel: w656 -> [w664 w668]
                    tunnel: w660 -> [_ w671]
                    tunnel: [w664 w665] -> w657
                    frame False {
                    }
                    frame True {
                      # "이거까지하면 1열 해결"
                      # "루프2단 시프트 레지스트 해서 해결"
                      # "2.3...돌떄 전에 돈값 가지고 돌아야 되는데"
                      # "이거 한번 돌면 한 열만 랭크한것"
                      n231 = Delete From Array(array=w668, index (row)=w671) -> (deleted portion=w670:dbl[])  [unwired: 2 in, 1 out]
                      n232 = Delete From Array(array=w668, index (row)=w666) -> (deleted portion=w669:dbl[])  [unwired: 2 in, 1 out]
                      n233 = Exclusive Or(1:w669, 2:w670) -> (0:w667:i32[])
                      n234 = Replace Array Subset(array=w668, new element=w667, index (row)=w666) -> (w665:dbl[][])  [unwired: 1 in]
                    }
                  }
                }
              }
            }
          }
        }
      }
      n235 = for {
        tunnel: w362 -> [w546] mode=indexing
        tunnel: [w545] -> w361 mode=indexing
        n236 = for {
          tunnel: w546 -> [w557] mode=indexing
          tunnel: [w556] -> w551 mode=indexing
          n237 = Reverse 1D Array(array=w557) -> (reversed array=w556:dbl[])
        }
        n238 = Array Size(array=w551) -> (size(s)=w550:i32[])
        n239 = Delete From Array(array=w550, index=1 ("인덱스")) -> (deleted portion=w548:i32)  [unwired: 1 in, 1 out]
        n240 = for {
          N: w548 -> [_]
          tunnel: w551 -> [w555]
          tunnel: [w552] -> w547 mode=indexing
          i -> [w554]
          n241 = Delete From Array(array=w555, index (col)=w554) -> (deleted portion=w553:dbl[])  [unwired: 2 in, 1 out]
          n242 = Reverse 1D Array(array=w553) -> (reversed array=w552:dbl[])
        }
        n243 = Transpose Matrix(1:w547) -> (0:w545:dbl[][])
      }
      n244 = for {
        tunnel: w361 -> [w432] mode=indexing
        tunnel: [w431] -> w360 mode=indexing
        n245 = Index Array(array=w432, index (row)=0 ("인덱스 (행)"), index (col)=0 ("인덱스 (열)")) -> (element=w435:dbl[][])
        n246 = Delete From Array(array=w435, index (col)=0 ("비활성화된 인덱스 (열)")) -> (deleted portion=w433:dbl[])  [unwired: 2 in, 1 out]
        n247 = for {
          tunnel: w433 -> [_] mode=indexing
          shift-right: [w448] -> w431
          shift-left: w432 -> [w441]
          i -> [w439]
          # "대각성분이 1일떄"
          n248 = Index Array(array=w441, index (row)=0 ("인덱스 (행)"), index (col)=0 ("인덱스 (열)")) -> (element=w443:dbl[][])
          n249 = Delete From Array(array=w443, index (col)=0 ("비활성화된 인덱스 (열)")) -> (deleted portion=w440:dbl[])  [unwired: 2 in, 1 out]
          n250 = Add(x=w439, y=1) -> (x+y=w447:i32)
          n251 = Delete From Array(array=w441, index (col)=w439) -> (deleted portion=w455:dbl[])  [unwired: 2 in, 1 out]
          n252 = Index Array(array=w440, index=w439) -> (element=w438:dbl)
          n253 = Equal?(x=w438, y=1.0) -> (x = y?=w450:bool)
          n254 = Split 1D Array(array=w455, index=w447) -> (second subarray=w451:dbl[])  [unwired: 1 out]
          n255 = call "Search Unsorted 1D Array.vim"("element"=1.0, "unsorted 1D array"=w451) -> ("index of element"=w453:i32)  [unwired: 9 in]
          n256 = Add(x=1, y=w453) -> (x+y=w446:i32)
          n257 = for {
            N: 1 -> [_]
            tunnel: w450 -> [w466]
            tunnel: w439 -> [w465]
            tunnel: w447 -> [w464]
            tunnel: w451 -> [w463]
            tunnel: w446 -> [w462]
            shift-right: [w461] -> w448
            shift-left: w441 -> [w460]
            tunnel: w439 -> [w459]
            tunnel: w447 -> [w458]
            n258 = case shown="True" w466 {
              tunnel: w463 -> [w475 w525]
              tunnel: w464 -> [w474 w527]
              tunnel: w460 -> [w471 w524]
              tunnel: w465 -> [w473 w526]
              tunnel: [w470 w523] -> w461
              tunnel: w465 -> [w472 _]
              tunnel: w462 -> [w469 _]
              tunnel: w459 -> [w468 _]
              tunnel: w458 -> [w467 _]
              frame False {
                n259 = for {
                  N: w469 -> [_]
                  tunnel: w475 -> [w484] mode=indexing
                  tunnel: w474 -> [w487]
                  tunnel: w473 -> [w485]
                  tunnel: w472 -> [w483]
                  shift-right: [w478] -> w470
                  shift-left: w471 -> [w479]
                  tunnel: w468 -> [w477]
                  tunnel: w467 -> [w476]
                  i -> [w480]
                  # "대각성분으로 넘어가야됨"
                  # "1처음나온거 바꾸고 그만해야됨"
                  n260 = Equal?(x=w484, y=1.0) -> (x = y?=w488:bool)
                  n261 = Add(x=w487, y=w480) -> (x+y=w486:i32)
                  n262 = Add(x=1, y=w480) -> (x+y=w481:i32)
                  n263 = case shown="True" w488 {
                    tunnel: w486 -> [_ w501]
                    tunnel: w485 -> [_ w503]
                    tunnel: w479 -> [w490 w505]
                    tunnel: w483 -> [_ w498]
                    tunnel: w481 -> [_ _]
                    tunnel: w477 -> [_ w492]
                    tunnel: [w490 w493] -> w478
                    tunnel: w476 -> [_ w491]
                    frame False {
                    }
                    frame True {
                      n264 = Delete From Array(array=w505, index (row)=w503) -> (deleted portion=w494:dbl[])  [unwired: 2 in, 1 out]
                      n265 = Delete From Array(array=w505, index (row)=w501) -> (deleted portion=w502:dbl[])  [unwired: 2 in, 1 out]
                      n266 = Replace Array Subset(array=w505, new element=w494, index (row)=w501) -> (w504:dbl[][])  [unwired: 1 in]
                      n267 = Replace Array Subset(array=w504, new element=w502, index (row)=w503) -> (w499:dbl[][])  [unwired: 1 in]
                      n268 = Delete From Array(array=w499, index (col)=w498) -> (deleted portion=w500:dbl[])  [unwired: 2 in, 1 out]
                      n269 = Add(x=w498, y=1) -> (x+y=w496:i32)
                      n270 = Split 1D Array(array=w500, index=w496) -> (second subarray=w495:dbl[])  [unwired: 1 out]
                      n271 = for {
                        tunnel: w495 -> [w508] mode=indexing
                        tunnel: w491 -> [w511]
                        tunnel: w492 -> [w509]
                        shift-right: [w507] -> w493
                        shift-left: w499 -> [w506]
                        i -> [w512]
                        n272 = Equal?(x=w508, y=1.0) -> (x = y?=w513:bool)
                        n273 = Add(x=w511, y=w512) -> (x+y=w510:i32)
                        n274 = case shown="True" w513 {
                          tunnel: w510 -> [_ w518]
                          tunnel: w509 -> [_ w522]
                          tunnel: w506 -> [w515 w519]
                          tunnel: [w515 w516] -> w507
                          frame False {
                          }
                          frame True {
                            # "32번안돌고 442 ,557번돔"
                            n275 = Delete From Array(array=w519, index (row)=w522) -> (deleted portion=w520:dbl[])  [unwired: 2 in, 1 out]
                            n276 = Delete From Array(array=w519, index (row)=w518) -> (deleted portion=w521:dbl[])  [unwired: 2 in, 1 out]
                            n277 = Exclusive Or(1:w521, 2:w520) -> (0:w517:i32[])
                            n278 = Replace Array Subset(array=w519, new element=w517, index (row)=w518) -> (w516:dbl[][])  [unwired: 1 in]
                          }
                        }
                      }
                    }
                  }
                }
              }
              frame True {
                n279 = for {
                  tunnel: w525 -> [w532] mode=indexing
                  tunnel: w527 -> [w535]
                  tunnel: w526 -> [w533]
                  shift-right: [w530] -> w523
                  shift-left: w524 -> [w529]
                  i -> [w536]
                  # "1열에서 1이 있는지"
                  n280 = Equal?(x=w532, y=1.0) -> (x = y?=w531:bool)
                  n281 = Add(x=w535, y=w536) -> (x+y=w534:i32)
                  n282 = case shown="True" w531 {
                    tunnel: w534 -> [_ w539]
                    tunnel: w529 -> [w537 w541]
                    tunnel: w533 -> [_ w544]
                    tunnel: [w537 w538] -> w530
                    frame False {
                    }
                    frame True {
                      # "이거까지하면 1열 해결"
                      # "루프2단 시프트 레지스트 해서 해결"
                      # "2.3...돌떄 전에 돈값 가지고 돌아야 되는데"
                      # "이거 한번 돌면 한 열만 랭크한것"
                      n283 = Delete From Array(array=w541, index (row)=w544) -> (deleted portion=w543:dbl[])  [unwired: 2 in, 1 out]
                      n284 = Delete From Array(array=w541, index (row)=w539) -> (deleted portion=w542:dbl[])  [unwired: 2 in, 1 out]
                      n285 = Exclusive Or(1:w542, 2:w543) -> (0:w540:i32[])
                      n286 = Replace Array Subset(array=w541, new element=w540, index (row)=w539) -> (w538:dbl[][])  [unwired: 1 in]
                    }
                  }
                }
              }
            }
          }
        }
      }
      n287 = for {
        tunnel: w360 -> [w419] mode=indexing
        tunnel: [w418] -> w359 mode=indexing
        n288 = for {
          tunnel: w419 -> [w430] mode=indexing
          tunnel: [w429] -> w424 mode=indexing
          n289 = Reverse 1D Array(array=w430) -> (reversed array=w429:dbl[])
        }
        n290 = Array Size(array=w424) -> (size(s)=w423:i32[])
        n291 = Delete From Array(array=w423, index=1 ("인덱스")) -> (deleted portion=w421:i32)  [unwired: 1 in, 1 out]
        n292 = for {
          N: w421 -> [_]
          tunnel: w424 -> [w428]
          tunnel: [w425] -> w420 mode=indexing
          i -> [w427]
          n293 = Delete From Array(array=w428, index (col)=w427) -> (deleted portion=w426:dbl[])  [unwired: 2 in, 1 out]
          n294 = Reverse 1D Array(array=w426) -> (reversed array=w425:dbl[])
        }
        n295 = Transpose Matrix(1:w420) -> (0:w418:dbl[][])
      }
      n296 = for {
        tunnel: w359 -> [w407] mode=indexing
        tunnel: [w406] -> w358 mode=indexing
        n297 = for {
          tunnel: w407 -> [w413] mode=indexing
          shift-right: [w409] -> w406
          shift-left: 0.0 -> [w408]
          n298 = Add Array Elements(numeric array=w413) -> (sum=w412:dbl)
          n299 = Greater Or Equal?(x=w412, y=1.0) -> (x >= y?=w410:bool)
          n300 = case shown="True" w410 {
            tunnel: [w414 w415] -> w409
            tunnel: w408 -> [w414 w417]
            frame False {
            }
            frame True {
              n301 = Add(x=w417, y=1.0) -> (x+y=w415:dbl)
            }
          }
        }
      }
      n302 = for {
        tunnel: w358 -> [w386] mode=indexing
        shift-right: [w382] -> w334
        shift-left: 0.0 -> [w381]
        shift-right: [w380] -> w333
        shift-left: 0.0 -> [w379]
        shift-right: [w378] -> w332
        shift-left: 0.0 -> [w377]
        n303 = Not Equal?(x=w386, y=32.0) -> (x != y?=w387:bool)
        n304 = Not Equal?(x=w386, y=31.0) -> (x != y?=w384:bool)
        n305 = Equal?(x=w386, y=32.0) -> (x = y?=w390:bool)
        n306 = Equal?(x=w386, y=31.0) -> (x = y?=w389:bool)
        n307 = And(x=w387, y=w384) -> (x .and. y?=w383:bool)
        n308 = case shown="True" w390 {
          tunnel: [w401 w404] -> w382
          tunnel: w381 -> [w401 w403]
          frame False {
          }
          frame True {
            n309 = Add(x=w403, y=1.0) -> (x+y=w404:dbl)
          }
        }
        n310 = case shown="True" w389 {
          tunnel: [w397 w399] -> w380
          tunnel: w379 -> [w397 w398]
          frame False {
          }
          frame True {
            n311 = Add(x=w398, y=1.0) -> (x+y=w399:dbl)
          }
        }
        n312 = case shown="True" w383 {
          tunnel: [w393 w396] -> w378
          tunnel: w377 -> [w393 w395]
          frame False {
          }
          frame True {
            n313 = Add(x=1.0, y=w395) -> (x+y=w396:dbl)
          }
        }
      }
      "32" <- w334
      "31" <- w333
      "0" <- w332
      n314 = Multiply(x=w331, y=0.2887880950866) -> (x*y=w350:dbl)
      n315 = Multiply(x=w331, y=0.5775761901732) -> (x*y=w348:dbl)
      n316 = Multiply(x=w331, y=0.1336357147402) -> (x*y=w346:dbl)
      n317 = Subtract(x=w334, y=w350) -> (x-y=w354:dbl)
      n318 = Subtract(x=w333, y=w348) -> (x-y=w353:dbl)
      n319 = Subtract(x=w332, y=w346) -> (x-y=w352:dbl)
      n320 = Square(x=w354) -> (x^2=w351:dbl)
      n321 = Square(x=w353) -> (x^2=w349:dbl)
      n322 = Square(x=w352) -> (x^2=w347:dbl)
      n323 = Divide(x=w351, y=w350) -> (x/y=w339:dbl)
      n324 = Divide(x=w349, y=w348) -> (x/y=w338:dbl)
      n325 = Divide(x=w347, y=w346) -> (x/y=w337:dbl)
      n326 = Compound Arithmetic op=ADD(w339, w338, w337) -> (w345:dbl)
      "X^2 2" <- w345
      n327 = Divide(x=w345, y=2.0) -> (x/y=w343:dbl)
      "결과" <- w343
      n328 = xnode "수식"("X1"=w343) -> ("결과"=w323:dbl)  [unwired: 1 in, 1 out]
      "?" <- w323
      n329 = Greater Or Equal?(x=w323, y=0.01) -> (x >= y?=w325:bool)
      n330 = case shown="False" w325 {
        tunnel: ["Failed" "Passed"] -> w324
        frame False {
        }
        frame True {
        }
      }
      "?" <- w324
    }
    frame #5 {
      n331 = Decimal String To Number(string=w692) -> (number=w723:i32[])  [unwired: 2 in, 1 out]
      n332 = Multiply(x=w723, y=2) -> (x*y=w721:i32[])
      n333 = Subtract(x=w721, y=1) -> (x-y=w694:i32[])
      n334 = call-poly <vilib>:"FFT.vi"("X"=w694) -> ("FFT {X}"=w698:cdb[])  [unwired: 9 in, 1 out]
      n335 = Complex To Polar(r * e^(i*theta)=w698) -> (r=w696:dbl[])  [unwired: 1 out]
      n336 = Array Size(array=w696) -> (size(s)=w695:i32)
      n337 = Array Size(array=w696) -> (size(s)=w719:i32)
      n338 = Divide(x=w719, y=2) -> (x/y=w693:dbl)
      n339 = Split 1D Array(array=w696, index=w693) -> (first subarray=w697:dbl[])  [unwired: 1 out]
      n340 = Natural Logarithm(1:20.0 ("x")) -> (0:w700:dbl)
      "log(x)" <- w700
      n341 = Multiply(x=w695, y=0.95) -> (x*y=w714:dbl)
      n342 = Multiply(x=w700, y=w695) -> (x*y=w717:dbl)
      n343 = Divide(x=w714, y=2.0) -> (x/y=w710:dbl)
      "N0" <- w710
      n344 = Square Root(x=w717) -> (sqrt(x)=→"T":dbl)
      n345 = for {
        tunnel: w697 -> [w730] mode=indexing
        shift-right: [w728] -> w711
        shift-left: 0.0 -> [w727]
        n346 = local read "T"() -> (w726:dbl)
        n347 = Less?(x=w730, y=w726) -> (x < y?=w729:bool)
        n348 = case shown="True" w729 {
          tunnel: [w731 w733] -> w728
          tunnel: w727 -> [w731 w732]
          frame False {
          }
          frame True {
            n349 = Add(x=w732, y=1.0) -> (x+y=w733:dbl)
          }
        }
      }
      "N1" <- w711
      n350 = Subtract(x=w711, y=w710) -> (x-y=w708:dbl)
      n351 = Multiply(x=w695, y=0.011875) -> (x*y=w709:dbl)
      n352 = Square Root(x=w709) -> (sqrt(x)=w707:dbl)
      n353 = Divide(x=w708, y=w707) -> (x/y=w706:dbl)
      "d" <- w706
      n354 = Absolute Value(x=w706) -> (abs(x)=w705:dbl)
      n355 = Square Root(x=2.0) -> (sqrt(x)=w703:dbl)
      n356 = Divide(x=w705, y=w703) -> (x/y=w702:dbl)
      "x" <- w702
      n357 = call <vilib>:"Error Function Complement.vi"("x"=w702) -> ("1 - erf(x)"=w688:dbl)  [unwired: 2 in]
      "1 - erf(x)" <- w688
      n358 = Greater Or Equal?(x=w688, y=0.01) -> (x >= y?=w690:bool)
      n359 = case shown="False" w690 {
        tunnel: ["Failed" "Passed"] -> w689
        frame False {
        }
        frame True {
        }
      }
      "?" <- w689
    }
    frame #6 {
      w741 = 8 ("y")
      n360 = Decimal String To Number(string=w739) -> (number=w742:i32[])  [unwired: 2 in, 1 out]
      n361 = Array Size(array=w742) -> (size(s)=w769:i32)
      n362 = Divide(x=w769, y=w741) -> (x/y=w768:dbl)
      n363 = Round Toward -Infinity(1:w768) -> (0:w740:dbl)
      "길이 M" <- w740
      n364 = Reshape Array(w742, w741, w740) -> (w767:i32[][])
      n365 = for {
        tunnel: w767 -> [w776] mode=indexing
        tunnel: [w775] -> w753 mode=indexing
        tunnel: [w773] -> w754
        n366 = Array Size(array=w776) -> (size(s)=w772:i32)
        n367 = for {
          N: w772 -> [_]
          shift-right: [w788] -> w775
          shift-left: 0.0 -> [w787]
          shift-right: [w785] -> _
          shift-left: w776 -> [w784]
          tunnel: [w777] -> w773
          i -> [w786]
          w778 = i32[] [0, 0, 0, 0, 0, 0, 0, 0, 1]
          n368 = Array Size(array=w778) -> (size(s)=w777:i32)
          n369 = Array Subset(array=w784, index=w786, length=w777) -> (w783:i32[])
          n370 = Array Size(array=w783) -> (size(s)=w782:i32)
          n371 = Equal?(x=w778, y=w783) -> (x = y?=w789:bool[])
          n372 = Equal?(x=w777, y=w782) -> (x = y?=w781:bool)
          n373 = And Array Elements(Boolean array=w789) -> (logical AND=w780:bool)
          n374 = And(x=w781, y=w780) -> (x .and. y?=w779:bool)
          n375 = case shown="True" w779 {
            tunnel: [w791 w801] -> w788
            tunnel: w787 -> [w791 w800]
            tunnel: w784 -> [w790 w799]
            tunnel: w786 -> [_ w797]
            tunnel: w777 -> [_ w794]
            tunnel: [w790 w798] -> w785
            frame False {
            }
            frame True {
              n376 = Add(x=w797, y=1) -> (x+y=w795:i32)
              n377 = Subtract(x=w794, y=1) -> (x-y=w792:i32)
              n378 = Add(x=w800, y=1.0) -> (x+y=w801:dbl)
              n379 = Delete From Array(array=w799, length=w792, index=w795) -> (array with subset deleted=w798:i32[])  [unwired: 1 out]
            }
          }
        }
      }
      n380 = Subtract(x=w740, y=w754) -> (x-y=w766:dbl)
      n381 = Power Of 2(x=w754) -> (2^x=w763:dbl)
      n382 = Add(x=w766, y=1) -> (x+y=w764:dbl)
      n383 = Multiply(x=w754, y=2.0) -> (x*y=w759:dbl)
      n384 = Divide(x=w764, y=w763) -> (x/y=w752:dbl)
      "u" <- w752
      n385 = Power Of 2(x=w759) -> (2^x=w758:dbl)
      n386 = Subtract(x=w759, y=1.0) -> (x-y=w760:dbl)
      n387 = Subtract(x=w753, y=w752) -> (x-y=w751:dbl[])
      n388 = Reciprocal(x=w763) -> (1/x=w757:dbl)
      n389 = Divide(x=w760, y=w758) -> (x/y=w756:dbl)
      n390 = Square(x=w751) -> (x^2=w750:dbl[])
      n391 = Add Array Elements(numeric array=w750) -> (sum=w749:dbl)
      n392 = Subtract(x=w757, y=w756) -> (x-y=w755:dbl)
      n393 = Multiply(x=w755, y=w740) -> (x*y=w748:dbl)
      "시그마^2" <- w748
      n394 = Divide(x=w749, y=w748) -> (x/y=w746:dbl)
      "X^2 3" <- w746
      n395 = Multiply(x=w746, y=0.5) -> (x*y=w743:dbl)
      n396 = Multiply(x=0.5, y=w741) -> (x*y=w744:dbl)
      n397 = call <vilib>:"Complementary Incomplete Gamma Function.vi"("a"=w743, "x"=w744) -> ("1 - g(x, a)"=w735:dbl)  [unwired: 1 in]
      "1 - g(x, a)" <- w735
      n398 = Greater Or Equal?(x=w735, y=0.01) -> (x >= y?=w737:bool)
      n399 = case shown="False" w737 {
        tunnel: ["Failed" "Passed"] -> w736
        frame False {
        }
        frame True {
        }
      }
      "?" <- w736
    }
    frame #7 {
      w808 = 1032 ("dimension size")
      (unwired) 0.138865
      (unwired) dbl[] [0.364091, 0.185659, 0.139381, 0.100571, 0.0704323, 0.139865] ("reversed array")
      (unwired) dbl[] [0.324652, 0.182617, 0.14267, 0.106645, 0.077147, 0.166269]
      # "m=LOG2 M"
      # "람다 에타 값에따라  파이값(0~5) 달라짐"
      n400 = Decimal String To Number(string=w807) -> (number=w867:i32[])  [unwired: 2 in, 1 out]
      n401 = Array Size(array=w867) -> (size(s)=w876:i32)
      n402 = Divide(x=w876, y=w808) -> (x/y=w875:dbl)
      n403 = Round Toward -Infinity(1:w875) -> (0:w853:dbl)
      n404 = Reshape Array(w867, w853, w808) -> (w874:i32[][])
      n405 = for {
        tunnel: w874 -> [w917] mode=indexing
        tunnel: [w920] -> w866 mode=indexing
        tunnel: [w918] -> w869
        n406 = Array Size(array=w917) -> (size(s)=w921:i32)
        n407 = for {
          N: w921 -> [_]
          shift-right: [w932] -> w920
          shift-left: 0.0 -> [w931]
          tunnel: [w924] -> w918
          tunnel: w917 -> [w923]
          i -> [w930]
          w922 = i32[] [1, 1, 1, 1, 1, 1, 1, 1, 1]
          n408 = Array Size(array=w922) -> (size(s)=w924:i32)
          n409 = Array Subset(array=w923, index=w930, length=w924) -> (w929:i32[])
          n410 = Array Size(array=w929) -> (size(s)=w928:i32)
          n411 = Equal?(x=w922, y=w929) -> (x = y?=w933:bool[])
          n412 = Equal?(x=w924, y=w928) -> (x = y?=w927:bool)
          n413 = And Array Elements(Boolean array=w933) -> (logical AND=w926:bool)
          n414 = And(x=w927, y=w926) -> (x .and. y?=w925:bool)
          n415 = case shown="True" w925 {
            tunnel: [w934 w936] -> w932
            tunnel: w931 -> [w934 w935]
            frame False {
            }
            frame True {
              n416 = Add(x=w935, y=1.0) -> (x+y=w936:dbl)
            }
          }
        }
      }
      n417 = for {
        tunnel: w866 -> [w888] mode=indexing
        tunnel: [w899] -> w865 mode=indexing
        tunnel: [w898] -> w864 mode=indexing
        tunnel: [w897] -> w863 mode=indexing
        tunnel: [w896] -> w862 mode=indexing
        tunnel: [w895] -> w861 mode=indexing
        tunnel: [w894] -> w860 mode=indexing
        n418 = Equal?(x=w888, y=0.0) -> (x = y?=w889:bool)
        n419 = Equal?(x=w888, y=1.0) -> (x = y?=w890:bool)
        n420 = Equal?(x=w888, y=2.0) -> (x = y?=w891:bool)
        n421 = Equal?(x=w888, y=3.0) -> (x = y?=w892:bool)
        n422 = Equal?(x=w888, y=4.0) -> (x = y?=w893:bool)
        n423 = Greater Or Equal?(x=w888, y=5.0) -> (x >= y?=w886:bool)
        n424 = case shown="True" w893 {
          tunnel: [0 1] -> w895
          frame False {
          }
          frame True {
          }
        }
        n425 = case shown="True" w886 {
          tunnel: [0 1] -> w894
          frame False {
          }
          frame True {
          }
        }
        n426 = case shown="True" w892 {
          tunnel: [0 1] -> w896
          frame False {
          }
          frame True {
          }
        }
        n427 = case shown="True" w891 {
          tunnel: [0 1] -> w897
          frame False {
          }
          frame True {
          }
        }
        n428 = case shown="True" w890 {
          tunnel: [0 1] -> w898
          frame False {
          }
          frame True {
          }
        }
        n429 = case shown="True" w889 {
          tunnel: [0 1] -> w899
          frame False {
          }
          frame True {
          }
        }
      }
      n430 = Subtract(x=w808, y=w869) -> (x-y=w873:i32)
      n431 = Power Of 2(x=w869) -> (2^x=w870:dbl)
      n432 = Add(x=w873, y=1) -> (x+y=w871:i32)
      n433 = Add Array Elements(numeric array=w861) -> (sum=w855:i32)
      "v4" <- w855
      n434 = Add Array Elements(numeric array=w860) -> (sum=w854:i32)
      "v5" <- w854
      n435 = Add Array Elements(numeric array=w863) -> (sum=w857:i32)
      "v2" <- w857
      n436 = Add Array Elements(numeric array=w862) -> (sum=w856:i32)
      "v3" <- w856
      n437 = Add Array Elements(numeric array=w864) -> (sum=w858:i32)
      "v1" <- w858
      n438 = Add Array Elements(numeric array=w865) -> (sum=w859:i32)
      "v0" <- w859
      n439 = Divide(x=w871, y=w870) -> (x/y=w847:dbl)
      "람다" <- w847
      n440 = Divide(x=w847, y=2.0) -> (x/y=w829:dbl)
      "에타" <- w829
      n441 = Build Array(w859, w858, w857, w856, w855, w854) -> (w852:i32[])
      n442 = Power Of X(1:w829, 2:3.0 ("y")) -> (0:w833:dbl)
      n443 = Square(x=w829) -> (x^2=w831:dbl)
      n444 = Divide(x=w833, y=24.0) -> (x/y=w823:dbl)
      n445 = Divide(x=w831, y=6.0) -> (x/y=w839:dbl)
      n446 = Divide(x=w831, y=2.0) -> (x/y=w824:dbl)
      n447 = Multiply(x=w829, y=3.0) -> (x*y=w827:dbl)
      n448 = Exponential(1:w829) -> (0:w846:dbl)
      n449 = Add(x=w829, y=w839) -> (x+y=w838:dbl)
      n450 = Divide(x=w827, y=2.0) -> (x/y=w825:dbl)
      n451 = Increment(x=w838) -> (x+1=w837:dbl)
      n452 = Multiply(x=w829, y=0.5) -> (x*y=w844:dbl)
      n453 = Reciprocal(x=w846) -> (1/x=w819:dbl)
      n454 = Compound Arithmetic op=ADD(w825, w824, w823) -> (w822:dbl)
      n455 = Increment(x=w822) -> (x+1=w820:dbl)
      n456 = Multiply(x=w819, y=w844) -> (x*y=w818:dbl)
      n457 = Multiply(x=w818, y=0.25) -> (x*y=w836:dbl)
      n458 = Add(x=w829, y=2.0) -> (x+y=w841:dbl)
      n459 = Multiply(x=w836, y=w837) -> (x*y=w816:dbl)
      n460 = Multiply(x=w836, y=w841) -> (x*y=w817:dbl)
      n461 = Multiply(x=w836, y=0.5) -> (x*y=w821:dbl)
      n462 = Multiply(x=w821, y=w820) -> (x*y=w815:dbl)
      n463 = Build Array(w819, w818, w817, w816, w815) -> (w812:dbl[])
      n464 = Add Array Elements(numeric array=w812) -> (sum=w813:dbl)
      n465 = Subtract(x=1.0, y=w813) -> (x-y=w811:dbl)
      n466 = Build Array (concatenate)(w812, w811) -> (w810:dbl[])
      n467 = for {
        tunnel: w853 -> [w884]
        tunnel: w810 -> [w885] mode=indexing
        tunnel: w852 -> [w883] mode=indexing
        tunnel: [w879] -> w851 mode=indexing
        n468 = Multiply(x=w885, y=w884) -> (x*y=w880:dbl)
        n469 = Subtract(x=w883, y=w880) -> (x-y=w882:dbl)
        n470 = Square(x=w882) -> (x^2=w881:dbl)
        n471 = Divide(x=w881, y=w880) -> (x/y=w879:dbl)
      }
      n472 = Add Array Elements(numeric array=w851) -> (sum=w848:dbl)
      "X^2 4" <- w848
      n473 = Divide(x=w848, y=2.0) -> (x/y=w849:dbl)
      n474 = call <vilib>:"Complementary Incomplete Gamma Function.vi"("a"=w849, "x"=2.5) -> ("1 - g(x, a)"=w803:dbl)  [unwired: 1 in]
      "P-VALUE 2" <- w803
      n475 = Greater Or Equal?(x=w803, y=0.01) -> (x >= y?=w805:bool)
      n476 = case shown="False" w805 {
        tunnel: ["Failed" "Passed"] -> w804
        frame False {
        }
        frame True {
        }
      }
      "?" <- w804
    }
    frame #8 {
      w952 = 496435200
      w957 = 231669760
      w960 = 107560960
      w963 = 49643520
      w966 = 22753280
      w969 = 10342400
      w972 = 4654080
      (unwired) enum16{"5120", "2560", "1280", "640", "1"}."5120"
      w975 = 2068480
      w990 = 904960
      w1053 = 387840
      # "K BIT"
      # "Q BIT"
      # "K BIT"
      # "Q BIT"
      n477 = Decimal String To Number(string=w983) -> (number=w1046:i32[])  [unwired: 2 in, 1 out]
      n478 = Array Size(array=w1046) -> (size(s)=w953:i32)
      n479 = Less?(x=w953, y=w975) -> (x < y?=w986:bool)
      n480 = Greater Or Equal?(x=w953, y=w990) -> (x >= y?=w985:bool)
      n481 = Less?(x=w953, y=w990) -> (x < y?=w988:bool)
      n482 = Less?(x=w953, y=w972) -> (x < y?=w978:bool)
      n483 = Greater Or Equal?(x=w953, y=w1053) -> (x >= y?=w989:bool)
      n484 = Less?(x=w953, y=w969) -> (x < y?=w974:bool)
      n485 = Greater Or Equal?(x=w953, y=w975) -> (x >= y?=w977:bool)
      n486 = Greater Or Equal?(x=w953, y=w972) -> (x >= y?=w973:bool)
      n487 = Less?(x=w953, y=w952) -> (x < y?=w959:bool)
      n488 = Less?(x=w953, y=1059061760) -> (x < y?=w956:bool)
      n489 = Less?(x=w953, y=w963) -> (x < y?=w968:bool)
      n490 = Less?(x=w953, y=w966) -> (x < y?=w971:bool)
      n491 = Greater Or Equal?(x=w953, y=w957) -> (x >= y?=w958:bool)
      n492 = Greater Or Equal?(x=w953, y=w952) -> (x >= y?=w955:bool)
      n493 = Greater Or Equal?(x=w953, y=w966) -> (x >= y?=w967:bool)
      n494 = Greater Or Equal?(x=w953, y=w969) -> (x >= y?=w970:bool)
      n495 = Less?(x=w953, y=w960) -> (x < y?=w965:bool)
      n496 = Less?(x=w953, y=w957) -> (x < y?=w962:bool)
      n497 = Greater Or Equal?(x=w953, y=w963) -> (x >= y?=w964:bool)
      n498 = Greater Or Equal?(x=w953, y=w960) -> (x >= y?=w961:bool)
      n499 = And(x=w985, y=w986) -> (x .and. y?=w984:bool)
      n500 = And(x=w989, y=w988) -> (x .and. y?=w987:bool)
      n501 = And(x=w977, y=w978) -> (x .and. y?=w976:bool)
      n502 = And(x=w973, y=w974) -> (x .and. y?=w951:bool)
      n503 = And(x=w958, y=w959) -> (x .and. y?=w946:bool)
      n504 = And(x=w955, y=w956) -> (x .and. y?=w945:bool)
      n505 = And(x=w967, y=w968) -> (x .and. y?=w949:bool)
      n506 = And(x=w970, y=w971) -> (x .and. y?=w950:bool)
      n507 = And(x=w964, y=w965) -> (x .and. y?=w948:bool)
      n508 = And(x=w961, y=w962) -> (x .and. y?=w947:bool)
      n509 = Less?(x=w953, y=w1053) -> (x < y?=w1052:bool)
      n510 = case shown="True" w1052 {
        tunnel: [0 ("y") 1 ("y")] -> w1051
        frame False {
        }
        frame True {
        }
      }
      n511 = case shown="True" w987 {
        tunnel: [0 ("y") 2 ("y")] -> w1050
        frame False {
        }
        frame True {
        }
      }
      n512 = case shown="True" w984 {
        tunnel: [0 ("y") 3 ("y")] -> w1049
        frame False {
        }
        frame True {
        }
      }
      n513 = case shown="True" w951 {
        tunnel: [0 ("y") 5 ("y")] -> w944
        frame False {
        }
        frame True {
        }
      }
      n514 = case shown="True" w976 {
        tunnel: [0 ("y") 4 ("y")] -> w1048
        frame False {
        }
        frame True {
        }
      }
      n515 = case shown="True" w950 {
        tunnel: [0 ("y") 6 ("y")] -> w943
        frame False {
        }
        frame True {
        }
      }
      n516 = case shown="True" w949 {
        tunnel: [0 ("y") 7 ("y")] -> w942
        frame False {
        }
        frame True {
        }
      }
      n517 = case shown="True" w948 {
        tunnel: [0 ("y") 8 ("y")] -> w941
        frame False {
        }
        frame True {
        }
      }
      n518 = case shown="True" w946 {
        tunnel: [0 ("y") 10 ("y")] -> w939
        frame False {
        }
        frame True {
        }
      }
      n519 = case shown="True" w947 {
        tunnel: [0 ("y") 9 ("y")] -> w940
        frame False {
        }
        frame True {
        }
      }
      n520 = case shown="True" w945 {
        tunnel: [0 ("y") 11 ("y")] -> w938
        frame False {
        }
        frame True {
        }
      }
      n521 = Compound Arithmetic op=ADD(w1051, w1050, w1049, w1048, w944, w943, w942, w941, w940, w939, w938) -> (w1047:i32)
      n522 = case shown="5" w1047 {
        tunnel: [9 ("y") 6 ("y") 6 ("y") 7 ("y") 8 ("y") 16 ("y") 10 ("y") 11 ("y") 12 ("y") 13 ("y") 14 ("y") 15 ("y")] -> w1019
        tunnel: [i32[][] array512x9[4608 elements] ("number") i32[][] [[0, 0, 0, 0, 0, 0], [0, 0, 0, 0, 0, 1], [0, 0, 0, 0, 1, 0], [0, 0, 0, 0, 1, 1], [0, 0, 0, 1, 0, 0], [0, 0, 0, 1, 0, 1], [0, 0, 0, 1, 1, 0], [0, 0, 0, 1, 1, 1], [0, 0, 1, 0, 0, 0], [0, 0, 1, 0, 0, 1], [0, 0, 1, 0, 1, 0], [0, 0, 1, 0, 1, 1], [0, 0, 1, 1, 0, 0], [0, 0, 1, 1, 0, 1], [0, 0, 1, 1, 1, 0], [0, 0, 1, 1, 1, 1], [0, 1, 0, 0, 0, 0], [0, 1, 0, 0, 0, 1], [0, 1, 0, 0, 1, 0], [0, 1, 0, 0, 1, 1], [0, 1, 0, 1, 0, 0], [0, 1, 0, 1, 0, 1], [0, 1, 0, 1, 1, 0], [0, 1, 0, 1, 1, 1], [0, 1, 1, 0, 0, 0], [0, 1, 1, 0, 0, 1], [0, 1, 1, 0, 1, 0], [0, 1, 1, 0, 1, 1], [0, 1, 1, 1, 0, 0], [0, 1, 1, 1, 0, 1], [0, 1, 1, 1, 1, 0], [0, 1, 1, 1, 1, 1], [1, 0, 0, 0, 0, 0], [1, 0, 0, 0, 0, 1], [1, 0, 0, 0, 1, 0], [1, 0, 0, 0, 1, 1], [1, 0, 0, 1, 0, 0], [1, 0, 0, 1, 0, 1], [1, 0, 0, 1, 1, 0], [1, 0, 0, 1, 1, 1], [1, 0, 1, 0, 0, 0], [1, 0, 1, 0, 0, 1], [1, 0, 1, 0, 1, 0], [1, 0, 1, 0, 1, 1], [1, 0, 1, 1, 0, 0], [1, 0, 1, 1, 0, 1], [1, 0, 1, 1, 1, 0], [1, 0, 1, 1, 1, 1], [1, 1, 0, 0, 0, 0], [1, 1, 0, 0, 0, 1], [1, 1, 0, 0, 1, 0], [1, 1, 0, 0, 1, 1], [1, 1, 0, 1, 0, 0], [1, 1, 0, 1, 0, 1], [1, 1, 0, 1, 1, 0], [1, 1, 0, 1, 1, 1], [1, 1, 1, 0, 0, 0], [1, 1, 1, 0, 0, 1], [1, 1, 1, 0, 1, 0], [1, 1, 1, 0, 1, 1], [1, 1, 1, 1, 0, 0], [1, 1, 1, 1, 0, 1], [1, 1, 1, 1, 1, 0], [1, 1, 1, 1, 1, 1]] ("출력 배열") i32[][] [[0, 0, 0, 0, 0, 0], [0, 0, 0, 0, 0, 1], [0, 0, 0, 0, 1, 0], [0, 0, 0, 0, 1, 1], [0, 0, 0, 1, 0, 0], [0, 0, 0, 1, 0, 1], [0, 0, 0, 1, 1, 0], [0, 0, 0, 1, 1, 1], [0, 0, 1, 0, 0, 0], [0, 0, 1, 0, 0, 1], [0, 0, 1, 0, 1, 0], [0, 0, 1, 0, 1, 1], [0, 0, 1, 1, 0, 0], [0, 0, 1, 1, 0, 1], [0, 0, 1, 1, 1, 0], [0, 0, 1, 1, 1, 1], [0, 1, 0, 0, 0, 0], [0, 1, 0, 0, 0, 1], [0, 1, 0, 0, 1, 0], [0, 1, 0, 0, 1, 1], [0, 1, 0, 1, 0, 0], [0, 1, 0, 1, 0, 1], [0, 1, 0, 1, 1, 0], [0, 1, 0, 1, 1, 1], [0, 1, 1, 0, 0, 0], [0, 1, 1, 0, 0, 1], [0, 1, 1, 0, 1, 0], [0, 1, 1, 0, 1, 1], [0, 1, 1, 1, 0, 0], [0, 1, 1, 1, 0, 1], [0, 1, 1, 1, 1, 0], [0, 1, 1, 1, 1, 1], [1, 0, 0, 0, 0, 0], [1, 0, 0, 0, 0, 1], [1, 0, 0, 0, 1, 0], [1, 0, 0, 0, 1, 1], [1, 0, 0, 1, 0, 0], [1, 0, 0, 1, 0, 1], [1, 0, 0, 1, 1, 0], [1, 0, 0, 1, 1, 1], [1, 0, 1, 0, 0, 0], [1, 0, 1, 0, 0, 1], [1, 0, 1, 0, 1, 0], [1, 0, 1, 0, 1, 1], [1, 0, 1, 1, 0, 0], [1, 0, 1, 1, 0, 1], [1, 0, 1, 1, 1, 0], [1, 0, 1, 1, 1, 1], [1, 1, 0, 0, 0, 0], [1, 1, 0, 0, 0, 1], [1, 1, 0, 0, 1, 0], [1, 1, 0, 0, 1, 1], [1, 1, 0, 1, 0, 0], [1, 1, 0, 1, 0, 1], [1, 1, 0, 1, 1, 0], [1, 1, 0, 1, 1, 1], [1, 1, 1, 0, 0, 0], [1, 1, 1, 0, 0, 1], [1, 1, 1, 0, 1, 0], [1, 1, 1, 0, 1, 1], [1, 1, 1, 1, 0, 0], [1, 1, 1, 1, 0, 1], [1, 1, 1, 1, 1, 0], [1, 1, 1, 1, 1, 1]] ("출력 배열") i32[][] [[0, 0, 0, 0, 0, 0, 0], [0, 0, 0, 0, 0, 0, 1], [0, 0, 0, 0, 0, 1, 0], [0, 0, 0, 0, 0, 1, 1], [0, 0, 0, 0, 1, 0, 0], [0, 0, 0, 0, 1, 0, 1], [0, 0, 0, 0, 1, 1, 0], [0, 0, 0, 0, 1, 1, 1], [0, 0, 0, 1, 0, 0, 0], [0, 0, 0, 1, 0, 0, 1], [0, 0, 0, 1, 0, 1, 0], [0, 0, 0, 1, 0, 1, 1], [0, 0, 0, 1, 1, 0, 0], [0, 0, 0, 1, 1, 0, 1], [0, 0, 0, 1, 1, 1, 0], [0, 0, 0, 1, 1, 1, 1], [0, 0, 1, 0, 0, 0, 0], [0, 0, 1, 0, 0, 0, 1], [0, 0, 1, 0, 0, 1, 0], [0, 0, 1, 0, 0, 1, 1], [0, 0, 1, 0, 1, 0, 0], [0, 0, 1, 0, 1, 0, 1], [0, 0, 1, 0, 1, 1, 0], [0, 0, 1, 0, 1, 1, 1], [0, 0, 1, 1, 0, 0, 0], [0, 0, 1, 1, 0, 0, 1], [0, 0, 1, 1, 0, 1, 0], [0, 0, 1, 1, 0, 1, 1], [0, 0, 1, 1, 1, 0, 0], [0, 0, 1, 1, 1, 0, 1], [0, 0, 1, 1, 1, 1, 0], [0, 0, 1, 1, 1, 1, 1], [0, 1, 0, 0, 0, 0, 0], [0, 1, 0, 0, 0, 0, 1], [0, 1, 0, 0, 0, 1, 0], [0, 1, 0, 0, 0, 1, 1], [0, 1, 0, 0, 1, 0, 0], [0, 1, 0, 0, 1, 0, 1], [0, 1, 0, 0, 1, 1, 0], [0, 1, 0, 0, 1, 1, 1], [0, 1, 0, 1, 0, 0, 0], [0, 1, 0, 1, 0, 0, 1], [0, 1, 0, 1, 0, 1, 0], [0, 1, 0, 1, 0, 1, 1], [0, 1, 0, 1, 1, 0, 0], [0, 1, 0, 1, 1, 0, 1], [0, 1, 0, 1, 1, 1, 0], [0, 1, 0, 1, 1, 1, 1], [0, 1, 1, 0, 0, 0, 0], [0, 1, 1, 0, 0, 0, 1], [0, 1, 1, 0, 0, 1, 0], [0, 1, 1, 0, 0, 1, 1], [0, 1, 1, 0, 1, 0, 0], [0, 1, 1, 0, 1, 0, 1], [0, 1, 1, 0, 1, 1, 0], [0, 1, 1, 0, 1, 1, 1], [0, 1, 1, 1, 0, 0, 0], [0, 1, 1, 1, 0, 0, 1], [0, 1, 1, 1, 0, 1, 0], [0, 1, 1, 1, 0, 1, 1], [0, 1, 1, 1, 1, 0, 0], [0, 1, 1, 1, 1, 0, 1], [0, 1, 1, 1, 1, 1, 0], [0, 1, 1, 1, 1, 1, 1], [1, 0, 0, 0, 0, 0, 0], [1, 0, 0, 0, 0, 0, 1], [1, 0, 0, 0, 0, 1, 0], [1, 0, 0, 0, 0, 1, 1], [1, 0, 0, 0, 1, 0, 0], [1, 0, 0, 0, 1, 0, 1], [1, 0, 0, 0, 1, 1, 0], [1, 0, 0, 0, 1, 1, 1], [1, 0, 0, 1, 0, 0, 0], [1, 0, 0, 1, 0, 0, 1], [1, 0, 0, 1, 0, 1, 0], [1, 0, 0, 1, 0, 1, 1], [1, 0, 0, 1, 1, 0, 0], [1, 0, 0, 1, 1, 0, 1], [1, 0, 0, 1, 1, 1, 0], [1, 0, 0, 1, 1, 1, 1], [1, 0, 1, 0, 0, 0, 0], [1, 0, 1, 0, 0, 0, 1], [1, 0, 1, 0, 0, 1, 0], [1, 0, 1, 0, 0, 1, 1], [1, 0, 1, 0, 1, 0, 0], [1, 0, 1, 0, 1, 0, 1], [1, 0, 1, 0, 1, 1, 0], [1, 0, 1, 0, 1, 1, 1], [1, 0, 1, 1, 0, 0, 0], [1, 0, 1, 1, 0, 0, 1], [1, 0, 1, 1, 0, 1, 0], [1, 0, 1, 1, 0, 1, 1], [1, 0, 1, 1, 1, 0, 0], [1, 0, 1, 1, 1, 0, 1], [1, 0, 1, 1, 1, 1, 0], [1, 0, 1, 1, 1, 1, 1], [1, 1, 0, 0, 0, 0, 0], [1, 1, 0, 0, 0, 0, 1], [1, 1, 0, 0, 0, 1, 0], [1, 1, 0, 0, 0, 1, 1], [1, 1, 0, 0, 1, 0, 0], [1, 1, 0, 0, 1, 0, 1], [1, 1, 0, 0, 1, 1, 0], [1, 1, 0, 0, 1, 1, 1], [1, 1, 0, 1, 0, 0, 0], [1, 1, 0, 1, 0, 0, 1], [1, 1, 0, 1, 0, 1, 0], [1, 1, 0, 1, 0, 1, 1], [1, 1, 0, 1, 1, 0, 0], [1, 1, 0, 1, 1, 0, 1], [1, 1, 0, 1, 1, 1, 0], [1, 1, 0, 1, 1, 1, 1], [1, 1, 1, 0, 0, 0, 0], [1, 1, 1, 0, 0, 0, 1], [1, 1, 1, 0, 0, 1, 0], [1, 1, 1, 0, 0, 1, 1], [1, 1, 1, 0, 1, 0, 0], [1, 1, 1, 0, 1, 0, 1], [1, 1, 1, 0, 1, 1, 0], [1, 1, 1, 0, 1, 1, 1], [1, 1, 1, 1, 0, 0, 0], [1, 1, 1, 1, 0, 0, 1], [1, 1, 1, 1, 0, 1, 0], [1, 1, 1, 1, 0, 1, 1], [1, 1, 1, 1, 1, 0, 0], [1, 1, 1, 1, 1, 0, 1], [1, 1, 1, 1, 1, 1, 0], [1, 1, 1, 1, 1, 1, 1]] ("출력 배열") i32[][] [[0, 0, 0, 0, 0, 0, 0, 0], [0, 0, 0, 0, 0, 0, 0, 1], [0, 0, 0, 0, 0, 0, 1, 0], [0, 0, 0, 0, 0, 0, 1, 1], [0, 0, 0, 0, 0, 1, 0, 0], [0, 0, 0, 0, 0, 1, 0, 1], [0, 0, 0, 0, 0, 1, 1, 0], [0, 0, 0, 0, 0, 1, 1, 1], [0, 0, 0, 0, 1, 0, 0, 0], [0, 0, 0, 0, 1, 0, 0, 1], [0, 0, 0, 0, 1, 0, 1, 0], [0, 0, 0, 0, 1, 0, 1, 1], [0, 0, 0, 0, 1, 1, 0, 0], [0, 0, 0, 0, 1, 1, 0, 1], [0, 0, 0, 0, 1, 1, 1, 0], [0, 0, 0, 0, 1, 1, 1, 1], [0, 0, 0, 1, 0, 0, 0, 0], [0, 0, 0, 1, 0, 0, 0, 1], [0, 0, 0, 1, 0, 0, 1, 0], [0, 0, 0, 1, 0, 0, 1, 1], [0, 0, 0, 1, 0, 1, 0, 0], [0, 0, 0, 1, 0, 1, 0, 1], [0, 0, 0, 1, 0, 1, 1, 0], [0, 0, 0, 1, 0, 1, 1, 1], [0, 0, 0, 1, 1, 0, 0, 0], [0, 0, 0, 1, 1, 0, 0, 1], [0, 0, 0, 1, 1, 0, 1, 0], [0, 0, 0, 1, 1, 0, 1, 1], [0, 0, 0, 1, 1, 1, 0, 0], [0, 0, 0, 1, 1, 1, 0, 1], [0, 0, 0, 1, 1, 1, 1, 0], [0, 0, 0, 1, 1, 1, 1, 1], [0, 0, 1, 0, 0, 0, 0, 0], [0, 0, 1, 0, 0, 0, 0, 1], [0, 0, 1, 0, 0, 0, 1, 0], [0, 0, 1, 0, 0, 0, 1, 1], [0, 0, 1, 0, 0, 1, 0, 0], [0, 0, 1, 0, 0, 1, 0, 1], [0, 0, 1, 0, 0, 1, 1, 0], [0, 0, 1, 0, 0, 1, 1, 1], [0, 0, 1, 0, 1, 0, 0, 0], [0, 0, 1, 0, 1, 0, 0, 1], [0, 0, 1, 0, 1, 0, 1, 0], [0, 0, 1, 0, 1, 0, 1, 1], [0, 0, 1, 0, 1, 1, 0, 0], [0, 0, 1, 0, 1, 1, 0, 1], [0, 0, 1, 0, 1, 1, 1, 0], [0, 0, 1, 0, 1, 1, 1, 1], [0, 0, 1, 1, 0, 0, 0, 0], [0, 0, 1, 1, 0, 0, 0, 1], [0, 0, 1, 1, 0, 0, 1, 0], [0, 0, 1, 1, 0, 0, 1, 1], [0, 0, 1, 1, 0, 1, 0, 0], [0, 0, 1, 1, 0, 1, 0, 1], [0, 0, 1, 1, 0, 1, 1, 0], [0, 0, 1, 1, 0, 1, 1, 1], [0, 0, 1, 1, 1, 0, 0, 0], [0, 0, 1, 1, 1, 0, 0, 1], [0, 0, 1, 1, 1, 0, 1, 0], [0, 0, 1, 1, 1, 0, 1, 1], [0, 0, 1, 1, 1, 1, 0, 0], [0, 0, 1, 1, 1, 1, 0, 1], [0, 0, 1, 1, 1, 1, 1, 0], [0, 0, 1, 1, 1, 1, 1, 1], [0, 1, 0, 0, 0, 0, 0, 0], [0, 1, 0, 0, 0, 0, 0, 1], [0, 1, 0, 0, 0, 0, 1, 0], [0, 1, 0, 0, 0, 0, 1, 1], [0, 1, 0, 0, 0, 1, 0, 0], [0, 1, 0, 0, 0, 1, 0, 1], [0, 1, 0, 0, 0, 1, 1, 0], [0, 1, 0, 0, 0, 1, 1, 1], [0, 1, 0, 0, 1, 0, 0, 0], [0, 1, 0, 0, 1, 0, 0, 1], [0, 1, 0, 0, 1, 0, 1, 0], [0, 1, 0, 0, 1, 0, 1, 1], [0, 1, 0, 0, 1, 1, 0, 0], [0, 1, 0, 0, 1, 1, 0, 1], [0, 1, 0, 0, 1, 1, 1, 0], [0, 1, 0, 0, 1, 1, 1, 1], [0, 1, 0, 1, 0, 0, 0, 0], [0, 1, 0, 1, 0, 0, 0, 1], [0, 1, 0, 1, 0, 0, 1, 0], [0, 1, 0, 1, 0, 0, 1, 1], [0, 1, 0, 1, 0, 1, 0, 0], [0, 1, 0, 1, 0, 1, 0, 1], [0, 1, 0, 1, 0, 1, 1, 0], [0, 1, 0, 1, 0, 1, 1, 1], [0, 1, 0, 1, 1, 0, 0, 0], [0, 1, 0, 1, 1, 0, 0, 1], [0, 1, 0, 1, 1, 0, 1, 0], [0, 1, 0, 1, 1, 0, 1, 1], [0, 1, 0, 1, 1, 1, 0, 0], [0, 1, 0, 1, 1, 1, 0, 1], [0, 1, 0, 1, 1, 1, 1, 0], [0, 1, 0, 1, 1, 1, 1, 1], [0, 1, 1, 0, 0, 0, 0, 0], [0, 1, 1, 0, 0, 0, 0, 1], [0, 1, 1, 0, 0, 0, 1, 0], [0, 1, 1, 0, 0, 0, 1, 1], [0, 1, 1, 0, 0, 1, 0, 0], [0, 1, 1, 0, 0, 1, 0, 1], [0, 1, 1, 0, 0, 1, 1, 0], [0, 1, 1, 0, 0, 1, 1, 1], [0, 1, 1, 0, 1, 0, 0, 0], [0, 1, 1, 0, 1, 0, 0, 1], [0, 1, 1, 0, 1, 0, 1, 0], [0, 1, 1, 0, 1, 0, 1, 1], [0, 1, 1, 0, 1, 1, 0, 0], [0, 1, 1, 0, 1, 1, 0, 1], [0, 1, 1, 0, 1, 1, 1, 0], [0, 1, 1, 0, 1, 1, 1, 1], [0, 1, 1, 1, 0, 0, 0, 0], [0, 1, 1, 1, 0, 0, 0, 1], [0, 1, 1, 1, 0, 0, 1, 0], [0, 1, 1, 1, 0, 0, 1, 1], [0, 1, 1, 1, 0, 1, 0, 0], [0, 1, 1, 1, 0, 1, 0, 1], [0, 1, 1, 1, 0, 1, 1, 0], [0, 1, 1, 1, 0, 1, 1, 1], [0, 1, 1, 1, 1, 0, 0, 0], [0, 1, 1, 1, 1, 0, 0, 1], [0, 1, 1, 1, 1, 0, 1, 0], [0, 1, 1, 1, 1, 0, 1, 1], [0, 1, 1, 1, 1, 1, 0, 0], [0, 1, 1, 1, 1, 1, 0, 1], [0, 1, 1, 1, 1, 1, 1, 0], [0, 1, 1, 1, 1, 1, 1, 1], [1, 0, 0, 0, 0, 0, 0, 0], [1, 0, 0, 0, 0, 0, 0, 1], [1, 0, 0, 0, 0, 0, 1, 0], [1, 0, 0, 0, 0, 0, 1, 1], [1, 0, 0, 0, 0, 1, 0, 0], [1, 0, 0, 0, 0, 1, 0, 1], [1, 0, 0, 0, 0, 1, 1, 0], [1, 0, 0, 0, 0, 1, 1, 1], [1, 0, 0, 0, 1, 0, 0, 0], [1, 0, 0, 0, 1, 0, 0, 1], [1, 0, 0, 0, 1, 0, 1, 0], [1, 0, 0, 0, 1, 0, 1, 1], [1, 0, 0, 0, 1, 1, 0, 0], [1, 0, 0, 0, 1, 1, 0, 1], [1, 0, 0, 0, 1, 1, 1, 0], [1, 0, 0, 0, 1, 1, 1, 1], [1, 0, 0, 1, 0, 0, 0, 0], [1, 0, 0, 1, 0, 0, 0, 1], [1, 0, 0, 1, 0, 0, 1, 0], [1, 0, 0, 1, 0, 0, 1, 1], [1, 0, 0, 1, 0, 1, 0, 0], [1, 0, 0, 1, 0, 1, 0, 1], [1, 0, 0, 1, 0, 1, 1, 0], [1, 0, 0, 1, 0, 1, 1, 1], [1, 0, 0, 1, 1, 0, 0, 0], [1, 0, 0, 1, 1, 0, 0, 1], [1, 0, 0, 1, 1, 0, 1, 0], [1, 0, 0, 1, 1, 0, 1, 1], [1, 0, 0, 1, 1, 1, 0, 0], [1, 0, 0, 1, 1, 1, 0, 1], [1, 0, 0, 1, 1, 1, 1, 0], [1, 0, 0, 1, 1, 1, 1, 1], [1, 0, 1, 0, 0, 0, 0, 0], [1, 0, 1, 0, 0, 0, 0, 1], [1, 0, 1, 0, 0, 0, 1, 0], [1, 0, 1, 0, 0, 0, 1, 1], [1, 0, 1, 0, 0, 1, 0, 0], [1, 0, 1, 0, 0, 1, 0, 1], [1, 0, 1, 0, 0, 1, 1, 0], [1, 0, 1, 0, 0, 1, 1, 1], [1, 0, 1, 0, 1, 0, 0, 0], [1, 0, 1, 0, 1, 0, 0, 1], [1, 0, 1, 0, 1, 0, 1, 0], [1, 0, 1, 0, 1, 0, 1, 1], [1, 0, 1, 0, 1, 1, 0, 0], [1, 0, 1, 0, 1, 1, 0, 1], [1, 0, 1, 0, 1, 1, 1, 0], [1, 0, 1, 0, 1, 1, 1, 1], [1, 0, 1, 1, 0, 0, 0, 0], [1, 0, 1, 1, 0, 0, 0, 1], [1, 0, 1, 1, 0, 0, 1, 0], [1, 0, 1, 1, 0, 0, 1, 1], [1, 0, 1, 1, 0, 1, 0, 0], [1, 0, 1, 1, 0, 1, 0, 1], [1, 0, 1, 1, 0, 1, 1, 0], [1, 0, 1, 1, 0, 1, 1, 1], [1, 0, 1, 1, 1, 0, 0, 0], [1, 0, 1, 1, 1, 0, 0, 1], [1, 0, 1, 1, 1, 0, 1, 0], [1, 0, 1, 1, 1, 0, 1, 1], [1, 0, 1, 1, 1, 1, 0, 0], [1, 0, 1, 1, 1, 1, 0, 1], [1, 0, 1, 1, 1, 1, 1, 0], [1, 0, 1, 1, 1, 1, 1, 1], [1, 1, 0, 0, 0, 0, 0, 0], [1, 1, 0, 0, 0, 0, 0, 1], [1, 1, 0, 0, 0, 0, 1, 0], [1, 1, 0, 0, 0, 0, 1, 1], [1, 1, 0, 0, 0, 1, 0, 0], [1, 1, 0, 0, 0, 1, 0, 1], [1, 1, 0, 0, 0, 1, 1, 0], [1, 1, 0, 0, 0, 1, 1, 1], [1, 1, 0, 0, 1, 0, 0, 0], [1, 1, 0, 0, 1, 0, 0, 1], [1, 1, 0, 0, 1, 0, 1, 0], [1, 1, 0, 0, 1, 0, 1, 1], [1, 1, 0, 0, 1, 1, 0, 0], [1, 1, 0, 0, 1, 1, 0, 1], [1, 1, 0, 0, 1, 1, 1, 0], [1, 1, 0, 0, 1, 1, 1, 1], [1, 1, 0, 1, 0, 0, 0, 0], [1, 1, 0, 1, 0, 0, 0, 1], [1, 1, 0, 1, 0, 0, 1, 0], [1, 1, 0, 1, 0, 0, 1, 1], [1, 1, 0, 1, 0, 1, 0, 0], [1, 1, 0, 1, 0, 1, 0, 1], [1, 1, 0, 1, 0, 1, 1, 0], [1, 1, 0, 1, 0, 1, 1, 1], [1, 1, 0, 1, 1, 0, 0, 0], [1, 1, 0, 1, 1, 0, 0, 1], [1, 1, 0, 1, 1, 0, 1, 0], [1, 1, 0, 1, 1, 0, 1, 1], [1, 1, 0, 1, 1, 1, 0, 0], [1, 1, 0, 1, 1, 1, 0, 1], [1, 1, 0, 1, 1, 1, 1, 0], [1, 1, 0, 1, 1, 1, 1, 1], [1, 1, 1, 0, 0, 0, 0, 0], [1, 1, 1, 0, 0, 0, 0, 1], [1, 1, 1, 0, 0, 0, 1, 0], [1, 1, 1, 0, 0, 0, 1, 1], [1, 1, 1, 0, 0, 1, 0, 0], [1, 1, 1, 0, 0, 1, 0, 1], [1, 1, 1, 0, 0, 1, 1, 0], [1, 1, 1, 0, 0, 1, 1, 1], [1, 1, 1, 0, 1, 0, 0, 0], [1, 1, 1, 0, 1, 0, 0, 1], [1, 1, 1, 0, 1, 0, 1, 0], [1, 1, 1, 0, 1, 0, 1, 1], [1, 1, 1, 0, 1, 1, 0, 0], [1, 1, 1, 0, 1, 1, 0, 1], [1, 1, 1, 0, 1, 1, 1, 0], [1, 1, 1, 0, 1, 1, 1, 1], [1, 1, 1, 1, 0, 0, 0, 0], [1, 1, 1, 1, 0, 0, 0, 1], [1, 1, 1, 1, 0, 0, 1, 0], [1, 1, 1, 1, 0, 0, 1, 1], [1, 1, 1, 1, 0, 1, 0, 0], [1, 1, 1, 1, 0, 1, 0, 1], [1, 1, 1, 1, 0, 1, 1, 0], [1, 1, 1, 1, 0, 1, 1, 1], [1, 1, 1, 1, 1, 0, 0, 0], [1, 1, 1, 1, 1, 0, 0, 1], [1, 1, 1, 1, 1, 0, 1, 0], [1, 1, 1, 1, 1, 0, 1, 1], [1, 1, 1, 1, 1, 1, 0, 0], [1, 1, 1, 1, 1, 1, 0, 1], [1, 1, 1, 1, 1, 1, 1, 0], [1, 1, 1, 1, 1, 1, 1, 1]] ("number") i32[][] array65536x16[1048576 elements] ("number") i32[][] array1024x10[10240 elements] ("number") i32[][] array2048x11[22528 elements] ("number") i32[][] array4096x12[49152 elements] ("number") i32[][] array8192x13[106496 elements] ("number") i32[][] array16384x14[229376 elements] ("number") i32[][] array32768x15[491520 elements] ("number")] -> w1034
        tunnel: [3.311 2.954 2.954 3.125 3.238 3.421 3.356 3.384 3.401 3.41 3.416 3.419] -> w1008
        tunnel: [8.1764248 5.2177052 5.2177052 6.1962507 7.1836656 15.167379 9.1723243 10.170032 11.168765 12.16807 13.167693 14.167488] -> w1003
        tunnel: [5120 ("y") 1 ("y") 640 1280 ("y") 2560 ("y") 655360 ("y") 10240 ("y") 20480 ("y") 40960 ("y") 81920 ("y") 163840 ("y") 327680 ("y")] -> w993
        frame 5 {
        }
        frame 1, Default {
          # "L-bit"
          # "variance"
          # "expected value"
        }
        frame 2 {
        }
        frame 3 {
        }
        frame 4 {
        }
        frame 0 {
        }
        frame 6 {
        }
        frame 7 {
        }
        frame 8 {
        }
        frame 9 {
        }
        frame 10 {
        }
        frame 11 {
        }
      }
      n523 = Divide(x=w953, y=w1019) -> (x/y=w1054:dbl)
      n524 = Round Toward -Infinity(1:w1054) -> (0:w1045:dbl)
      n525 = Reshape Array(w1046, w1045, w1019) -> (w1040:i32[][])
      n526 = case shown="0, Default" w993 {
        tunnel: w1040 -> [w1075 w1079 w1083 w1087 w1091 w1094 w1099 w1103 w1107 w1111 w1115 w1119]
        tunnel: [w1073 w1078 w1082 w1086 w1090 w1095 w1098 w1102 w1106 w1110 w1114 w1118] -> w1037
        tunnel: [w1071 w1081 w1085 w1089 w1093 w1096 w1100 w1104 w1108 w1112 w1116 w1120] -> w992
        tunnel: w993 -> [_ w1081 w1085 w1089 w1093 w1096 w1100 w1104 w1108 w1112 w1116 w1120]
        frame 0, Default {
          n527 = Array Size(array=w1075) -> (size(s)=w1074:i32[])
          n528 = Array Max & Min(array=w1074) -> (max value=w1073:i32)  [unwired: 3 out]
          n529 = Divide(x=w1073, y=101) -> (x/y=w1076:dbl)
          n530 = Round To Nearest(number=w1076) -> (nearest integer value=w1072:dbl)
          n531 = To Long Integer(number=w1072) -> (32bit integer=w1071:i32)
        }
        frame 640 {
          n532 = Array Size(array=w1079) -> (size(s)=w1080:i32[])
          n533 = Array Max & Min(array=w1080) -> (max value=w1078:i32)  [unwired: 3 out]
        }
        frame 1280 {
          n534 = Array Size(array=w1083) -> (size(s)=w1084:i32[])
          n535 = Array Max & Min(array=w1084) -> (max value=w1082:i32)  [unwired: 3 out]
        }
        frame 2560 {
          n536 = Array Size(array=w1087) -> (size(s)=w1088:i32[])
          n537 = Array Max & Min(array=w1088) -> (max value=w1086:i32)  [unwired: 3 out]
        }
        frame 5120 {
          n538 = Array Size(array=w1091) -> (size(s)=w1092:i32[])
          n539 = Array Max & Min(array=w1092) -> (max value=w1090:i32)  [unwired: 3 out]
        }
        frame 10240 {
          n540 = Array Size(array=w1094) -> (size(s)=w1097:i32[])
          n541 = Array Max & Min(array=w1097) -> (max value=w1095:i32)  [unwired: 3 out]
        }
        frame 20480 {
          n542 = Array Size(array=w1099) -> (size(s)=w1101:i32[])
          n543 = Array Max & Min(array=w1101) -> (max value=w1098:i32)  [unwired: 3 out]
        }
        frame 40960 {
          n544 = Array Size(array=w1103) -> (size(s)=w1105:i32[])
          n545 = Array Max & Min(array=w1105) -> (max value=w1102:i32)  [unwired: 3 out]
        }
        frame 81920 {
          n546 = Array Size(array=w1107) -> (size(s)=w1109:i32[])
          n547 = Array Max & Min(array=w1109) -> (max value=w1106:i32)  [unwired: 3 out]
        }
        frame 163840 {
          n548 = Array Size(array=w1111) -> (size(s)=w1113:i32[])
          n549 = Array Max & Min(array=w1113) -> (max value=w1110:i32)  [unwired: 3 out]
        }
        frame 327680 {
          n550 = Array Size(array=w1115) -> (size(s)=w1117:i32[])
          n551 = Array Max & Min(array=w1117) -> (max value=w1114:i32)  [unwired: 3 out]
        }
        frame 655360 {
          n552 = Array Size(array=w1119) -> (size(s)=w1121:i32[])
          n553 = Array Max & Min(array=w1121) -> (max value=w1118:i32)  [unwired: 3 out]
        }
      }
      n554 = Subtract(x=w1019, y=1) -> (x-y=w1038:i32)
      n555 = Subtract(x=w1037, y=1) -> (x-y=w1035:i32)
      n556 = Decrement(x=w992) -> (x-1=w991:i32)
      n557 = Add(x=w991, y=1) -> (x+y=w1033:i32)
      n558 = Array Subset(array=w1040, index (row)=0 ("행 1"), length (row)=w991, index (col)=0 ("열 1"), length (col)=w1038) -> (w995:dbl[][])
      n559 = Array Subset(array=w1040, index (row)=w1033, length (row)=w1035, index (col)=0 ("열 1"), length (col)=w1038) -> (w994:dbl[][])
      n560 = for {
        tunnel: w995 -> [w1151] mode=indexing
        tunnel: w1034 -> [w1150]
        tunnel: [w1149] -> w1032 mode=indexing
        n561 = while {
          tunnel: w1150 -> [w1155] mode=indexing
          tunnel: w1151 -> [w1156]
          tunnel: [w1152] -> w1149
          i -> [w1152]
          stop <- w1153 stop-if-true
          n562 = Equal?(x=w1155, y=w1156) -> (x = y?=w1154:bool[])
          n563 = And Array Elements(Boolean array=w1154) -> (logical AND=w1153:bool)
        }
      }
      n564 = for {
        tunnel: w994 -> [w1143] mode=indexing
        tunnel: w1034 -> [w1142]
        tunnel: [w1141] -> w1030 mode=indexing
        n565 = while {
          tunnel: w1142 -> [w1147] mode=indexing
          tunnel: w1143 -> [w1148]
          tunnel: [w1144] -> w1141
          i -> [w1144]
          stop <- w1145 stop-if-true
          n566 = Equal?(x=w1147, y=w1148) -> (x = y?=w1146:bool[])
          n567 = And Array Elements(Boolean array=w1146) -> (logical AND=w1145:bool)
        }
      }
      n568 = Array Size(array=w1032) -> (size(s)=w1031:i32)
      n569 = Array Size(array=w1030) -> (size(s)=w1009:i32)
      n570 = Insert Into Array(array=w1032, index=w1031, new element=w1030) -> (w1029:i32[])
      n571 = for {
        N: w1009 -> [_]
        tunnel: w1029 -> [w1138]
        tunnel: w1033 -> [w1134]
        tunnel: [w1132] -> w1028 mode=indexing
        i -> [w1133]
        n572 = Add(x=w1133, y=w1134) -> (x+y=w1122:i32)
        n573 = Index Array(array=w1138, index=w1122) -> (element=w1135:i32)
        n574 = Array Subset(array=w1138, index=0 ("인덱스"), length=w1122) -> (w1131:i32[])
        n575 = Add(x=w1122, y=1) -> (x+y=w1124:i32)
        n576 = Reverse 1D Array(array=w1131) -> (reversed array=w1136:i32[])
        n577 = call "Search Unsorted 1D Array.vim"("element"=w1135, "unsorted 1D array"=w1136) -> ("index of element"=w1127:i32)  [unwired: 9 in]
        n578 = Array Size(array=w1131) -> (size(s)=w1123:i32)
        n579 = Equal?(x=w1127, y=-1 ("index of element")) -> (x = y?=w1128:bool)
        n580 = case shown="True" w1128 {
          tunnel: [w1139 w1140] -> w1126
          tunnel: w1127 -> [w1139 _]
          tunnel: w1123 -> [_ w1140]
          frame False {
          }
          frame True {
          }
        }
        n581 = Subtract(x=w1123, y=w1126) -> (x-y=w1130:i32)
        n582 = Subtract(x=w1124, y=w1130) -> (x-y=w1132:i32)
      }
      n583 = Divide(x=0.8, y=w1019) -> (x/y=w1011:dbl)
      n584 = Subtract(x=0.7, y=w1011) -> (x-y=w1010:dbl)
      n585 = Divide(x=32.0, y=w1019) -> (x/y=w1021:dbl)
      n586 = Logarithm Base 2(1:w1028) -> (0:w1027:dbl[])
      n587 = Add(x=4.0, y=w1021) -> (x+y=w1013:dbl)
      n588 = Add Array Elements(numeric array=w1027) -> (sum=w1026:dbl)
      n589 = Divide(x=w1026, y=w1009) -> (x/y=w1004:dbl)
      "f(n)" <- w1004
      n590 = Divide(x=3.0, y=w1019) -> (x/y=w1018:dbl)
      n591 = Negate(x=w1018) -> (-x=w1017:dbl)
      n592 = Power Of X(1:w1009, 2:w1017) -> (0:w1016:dbl)
      n593 = Divide(x=w1016, y=15.0) -> (x/y=w1014:dbl)
      n594 = Multiply(x=w1014, y=w1013) -> (x*y=w1012:dbl)
      n595 = Subtract(x=w1004, y=w1003) -> (x-y=w1002:dbl)
      n596 = Add(x=w1010, y=w1012) -> (x+y=w1005:dbl)
      "c" <- w1005
      n597 = Divide(x=w1008, y=w1009) -> (x/y=w1007:dbl)
      n598 = Square Root(x=w1007) -> (sqrt(x)=w1006:dbl)
      n599 = Square Root(x=2.0) -> (sqrt(x)=w1000:dbl)
      n600 = Multiply(x=w1005, y=w1006) -> (x*y=w999:dbl)
      "시그마" <- w999
      n601 = Multiply(x=w1000, y=w999) -> (x*y=w998:dbl)
      n602 = Divide(x=w1002, y=w998) -> (x/y=w997:dbl)
      n603 = Absolute Value(x=w997) -> (abs(x)=w996:dbl)
      "erfc( )" <- w996
      n604 = call <vilib>:"Error Function Complement.vi"("x"=w996) -> ("1 - erf(x)"=w979:dbl)  [unwired: 2 in]
      "p-value 4" <- w979
      n605 = Greater Or Equal?(x=w979, y=0.01) -> (x >= y?=w981:bool)
      n606 = case shown="False" w981 {
        tunnel: ["Failed" "Passed"] -> w980
        frame False {
        }
        frame True {
        }
      }
      "?" <- w980
    }
    frame #9 {
      (unwired) dbl[] [0.010417, 0.03125, 0.125, 0.5, 0.25, 0.0625, 0.020833]
      # "합 1.~5"
      # "합 1인건데 이거안씀"
      # "x^2"
      # "u"
      n607 = Equal?(x="dimension size", y=0) -> (x = y?=w1227:bool)
      n608 = Decimal String To Number(string=w1233) -> (number=w1284:i32[])  [unwired: 2 in, 1 out]
      n609 = case shown="True" w1227 {
        tunnel: [w1285 500] -> w1225
        tunnel: "dimension size" -> [w1285 _]
        frame False {
        }
        frame True {
        }
      }
      n610 = Array Size(array=w1284) -> (size(s)=w1283:i32)
      n611 = Divide(x=w1283, y=w1225) -> (x/y=w1236:dbl)
      n612 = Round Toward -Infinity(1:w1236) -> (0:w1235:dbl)
      n613 = Reshape Array(w1284, w1235, w1225) -> (w1237:i32[][])
      n614 = for {
        tunnel: [w1349] -> w1238 mode=indexing
        tunnel: [w1347] -> _ mode=indexing
        tunnel: w1237 -> [w1347] mode=indexing
        (unwired) i32[] [1, 1, 0, 1, 0, 1, 1, 1, 1, 0, 0, 0, 1]
        (unwired) i32[] [0, 1, 1, 1, 0, 1, 1, 0, 0, 0]
        (unwired) i32[] [1, 0, 0, 1, 0, 0, 1, 1, 1, 1, 1]
        (unwired) i32[] [1, 0, 1, 0, 1, 0, 1, 0, 0, 1, 1, 0, 0, 1]
        # "길이 4"
        # "3"
        # "2"
        # "1"
        # "h(x)"
        # "g(x)"
        # "이전 b(j)"
        # "이전 m(j)"
        # "G(x)의 첫쨰값"
        n615 = Index Array(array=w1347, index=0) -> (element=w1348:i32)
        n616 = while {
          shift-right: [w1371] -> _
          shift-left: 0 -> [w1405]
          shift-right: [w1389] -> _
          shift-left: w1348 -> [w1394]
          shift-right: [w1357] -> _
          shift-left: i32[] [1] ("Numeric") -> [w1395]
          shift-right: [w1398] -> _
          shift-left: i32[] [0, 1] ("Numeric") -> [w1404]
          tunnel: w1347 -> [w1370]
          tunnel: w1347 -> [w1369]
          tunnel: [w1357] -> _ mode=indexing
          tunnel: [w1356] -> w1349
          i -> [w1390]
          stop <- w1384 stop-if-true
          w1380 = -0.5
          w1408 = 0 ("y")
          # "(x^k)*g(1/x)"
          # "x^k"
          # "b(j)"
          # "b*x*g(x)에서 b1이라 안곱해도상관x"
          n617 = Multiply(x=w1404, y=w1394) -> (x*y=w1403:i32[])
          n618 = Build Array(w1395, w1403) -> (w1396:i32[][])
          n619 = Index Array(array=w1396, index (row)=0) -> (element=w1399:i32[])  [unwired: 1 in]
          n620 = Index Array(array=w1396, index (row)=1) -> (element=w1400:i32[])  [unwired: 1 in]
          n621 = Greater Or Equal?(x=w1405, y=w1408) -> (x >= y?=w1407:bool)
          n622 = Not Equal?(x=w1408, y=w1394) -> (x != y?=w1406:bool)
          n623 = And(x=w1407, y=w1406) -> (x .and. y?=w1397:bool)
          n624 = Exclusive Or(1:w1400, 2:w1399) -> (0:w1357:i32[])
          n625 = case shown="False" w1397 {
            tunnel: w1405 -> [w1469 w1488]
            tunnel: [w1468 w1487] -> w1371
            tunnel: w1395 -> [_ w1483]
            tunnel: w1404 -> [w1464 _]
            tunnel: [w1463 w1482] -> w1398
            frame False {
              # "x"
              n626 = Increment(x=w1469) -> (x+1=w1468:i32)
              n627 = for {
                tunnel: i32[] [0, 1] ("Numeric") -> [w1478] mode=indexing
                tunnel: [w1473] -> w1466 mode=indexing
                tunnel: w1464 -> [w1472]
                i -> [w1476]
                w1474 = 0 ("Numeric")
                # "g(x)"
                n628 = for {
                  tunnel: w1478 -> [w1481]
                  tunnel: [w1480] -> w1477 mode=indexing
                  tunnel: w1472 -> [w1479] mode=indexing
                  n629 = Multiply(x=w1479, y=w1481) -> (x*y=w1480:i32)
                }
                n630 = Initialize Array(w1474, w1476) -> (w1475:i32[])
                n631 = Insert Into Array(array=w1477, index=w1474, new element=w1475) -> (w1473:i32[])
              }
              n632 = Transpose 2D Array(2D array=w1466) -> (transposed array=w1467:i32[][])
              n633 = for {
                tunnel: w1467 -> [w1471] mode=indexing
                tunnel: [w1470] -> w1463 mode=indexing
                n634 = Add Array Elements(numeric array=w1471) -> (sum=w1470:i32)
              }
            }
            frame True {
              # "x"
              n635 = Negate(x=w1488) -> (-x=w1487:i32)
              n636 = for {
                tunnel: i32[] [0, 1] ("Numeric") -> [w1497] mode=indexing
                tunnel: [w1492] -> w1485 mode=indexing
                tunnel: w1483 -> [w1491]
                i -> [w1495]
                w1493 = 0 ("Numeric")
                # "g(x)"
                n637 = for {
                  tunnel: w1491 -> [w1499] mode=indexing
                  tunnel: w1497 -> [w1500]
                  tunnel: [w1498] -> w1496 mode=indexing
                  n638 = Multiply(x=w1499, y=w1500) -> (x*y=w1498:i32)
                }
                n639 = Initialize Array(w1493, w1495) -> (w1494:i32[])
                n640 = Insert Into Array(array=w1496, index=w1493, new element=w1494) -> (w1492:i32[])
              }
              n641 = Transpose 2D Array(2D array=w1485) -> (transposed array=w1486:i32[][])
              n642 = for {
                tunnel: w1486 -> [w1490] mode=indexing
                tunnel: [w1489] -> w1482 mode=indexing
                n643 = Add Array Elements(numeric array=w1490) -> (sum=w1489:i32)
              }
            }
          }
          n644 = for {
            tunnel: w1357 -> [w1459] mode=indexing
            tunnel: [w1454] -> w1392 mode=indexing
            tunnel: w1369 -> [w1453]
            i -> [w1457]
            w1455 = 0 ("Numeric")
            # "G(x)"
            n645 = for {
              tunnel: w1453 -> [w1461] mode=indexing
              tunnel: w1459 -> [w1462]
              tunnel: [w1460] -> w1458 mode=indexing
              n646 = Multiply(x=w1461, y=w1462) -> (x*y=w1460:i32)
            }
            n647 = Initialize Array(w1455, w1457) -> (w1456:i32[])
            n648 = Insert Into Array(array=w1458, index=w1455, new element=w1456) -> (w1454:i32[])
          }
          n649 = Increment(x=w1390) -> (x+1=w1379:i32)
          n650 = Transpose 2D Array(2D array=w1392) -> (transposed array=w1393:i32[][])
          n651 = for {
            tunnel: w1393 -> [w1452] mode=indexing
            tunnel: [w1449] -> w1391 mode=indexing
            n652 = Add Array Elements(numeric array=w1452) -> (sum=w1451:i32)
            n653 = Quotient & Remainder(x=w1451, y=2) -> (x-y*floor(x/y)=w1449:i32)  [unwired: 1 out]
          }
          n654 = Index Array(array=w1391, index=w1379) -> (element=w1389:i32)
          n655 = Multiply(x=w1380, y=w1371) -> (x*y=w1381:dbl)
          n656 = Negate(x=w1380) -> (-x=w1378:dbl)
          n657 = Add(x=w1378, y=w1381) -> (x+y=w1377:dbl)
          n658 = Multiply(x=w1379, y=w1378) -> (x*y=w1376:dbl)
          n659 = Add(x=w1376, y=w1377) -> (x+y=w1355:dbl)
          n660 = Round Toward -Infinity(1:w1355) -> (0:w1354:dbl)
          n661 = Initialize Array(0, w1354) -> (w1360:i32[])
          n662 = Insert Into Array(array=w1360, new element=1 ("new element/subarray")) -> (w1359:i32[])  [unwired: 1 in]
          n663 = for {
            tunnel: w1359 -> [w1420] mode=indexing
            tunnel: [w1413] -> w1372 mode=indexing
            tunnel: w1357 -> [w1415]
            i -> [w1418]
            # "G(x)"
            n664 = Array Size(array=w1415) -> (size(s)=w1419:i32)
            n665 = Decrement(x=w1419) -> (x-1=w1414:i32)
            n666 = Initialize Array(0 ("element"), w1414) -> (w1416:i32[])
            n667 = for {
              tunnel: w1415 -> [w1427] mode=indexing
              tunnel: w1420 -> [w1428]
              tunnel: w1418 -> [w1426]
              shift-right: [w1422] -> w1413
              shift-left: w1416 -> [w1421]
              i -> [w1425]
              n668 = Subtract(x=w1426, y=w1425) -> (x-y=w1423:i32)
              n669 = Multiply(x=w1427, y=w1428) -> (x*y=w1424:i32)
              n670 = Replace Array Subset(array=w1421, new element=w1424, index=w1423) -> (w1422:i32[])
            }
          }
          n671 = Transpose 2D Array(2D array=w1372) -> (transposed array=w1373:i32[][])
          n672 = for {
            tunnel: w1373 -> [w1412] mode=indexing
            tunnel: [w1409] -> w1358 mode=indexing
            n673 = Add Array Elements(numeric array=w1412) -> (sum=w1411:i32)
            n674 = Quotient & Remainder(x=w1411, y=2) -> (x-y*floor(x/y)=w1409:i32)  [unwired: 1 out]
          }
          n675 = Reverse 1D Array(array=w1358) -> (reversed array=w1387:i32[])
          n676 = call "Search Unsorted 1D Array.vim"("element"=1.0, "unsorted 1D array"=w1387) -> ("index of element"=w1386:i32)  [unwired: 9 in]
          n677 = Increment(x=w1386) -> (x+1=w1385:i32)
          n678 = Split 1D Array(array=w1387, index=w1385) -> (second subarray=w1383:i32[])  [unwired: 1 out]
          n679 = Reverse 1D Array(array=w1383) -> (reversed array=w1367:i32[])
          n680 = Reverse 1D Array(array=w1358) -> (reversed array=w1365:i32[])
          n681 = Array Size(array=w1367) -> (size(s)=w1368:i32)
          n682 = call "Search Unsorted 1D Array.vim"("element"=1.0, "unsorted 1D array"=w1365) -> ("index of element"=w1364:i32)  [unwired: 9 in]
          n683 = Split 1D Array(array=w1365, index=w1364) -> (second subarray=w1363:i32[])  [unwired: 1 out]
          n684 = while {
            tunnel: w1368 -> [w1442]
            tunnel: w1367 -> [w1443]
            tunnel: [w1435] -> w1382 mode=indexing
            tunnel: w1370 -> [w1429]
            i -> [w1430]
            stop <- w1432 stop-if-true
            n685 = Add(x=w1442, y=w1430) -> (x+y=w1431:i32)
            n686 = Array Subset(array=w1429, index=w1430, length=w1442) -> (w1444:i32[])
            n687 = Array Size(array=w1429) -> (size(s)=w1434:i32)
            n688 = Index Array(array=w1429, index=w1431) -> (element=w1436:i32)
            n689 = Decrement(x=w1434) -> (x-1=w1433:i32)
            n690 = Equal?(x=w1433, y=w1431) -> (x = y?=w1432:bool)
            n691 = Multiply(x=w1444, y=w1443) -> (x*y=w1441:i32[])
            n692 = Delete From Array(array=w1441, index=0) -> (deleted portion=w1439:i32, array with subset deleted=w1438:i32[])  [unwired: 1 in]
            n693 = for {
              tunnel: w1438 -> [w1448] mode=indexing
              shift-right: [w1445] -> w1437
              shift-left: w1439 -> [w1447]
              n694 = Not Equal?(x=w1447, y=w1448) -> (x != y?=w1446:bool)
              n695 = Boolean To (0,1)(Boolean=w1446) -> (0, 1=w1445:i16)
            }
            n696 = Equal?(x=w1437, y=w1436) -> (x = y?=w1435:bool)
          }
          n697 = Reverse 1D Array(array=w1363) -> (reversed array=w1362:i32[])
          n698 = Array Size(array=w1362) -> (size(s)=w1361:i32)
          n699 = Decrement(x=w1361) -> (x-1=w1356:i32)
          n700 = And Array Elements(Boolean array=w1382) -> (logical AND=w1384:bool)
        }
      }
      n701 = Divide(x=w1225, y=3.0) -> (x/y=w1274:dbl)
      n702 = Divide(x=2.0, y=9.0) -> (x/y=w1271:dbl)
      n703 = Increment(x=w1225) -> (x+1=w1280:i32)
      n704 = Add(x=w1274, y=w1271) -> (x+y=w1270:dbl)
      n705 = Power Of X(1:-1.0 ("x"), 2:w1280) -> (0:w1279:dbl)
      n706 = Power Of 2(x=w1225) -> (2^x=w1269:dbl)
      n707 = Divide(x=w1270, y=w1269) -> (x/y=w1268:dbl)
      n708 = Add(x=w1279, y=9.0) -> (x+y=w1277:dbl)
      n709 = Negate(x=w1268) -> (-x=w1265:dbl)
      n710 = Multiply(x=0.5 ("y"), y=w1225) -> (x*y=w1267:dbl)
      n711 = Divide(x=w1277, y=36.0) -> (x/y=w1266:dbl)
      n712 = Compound Arithmetic op=ADD(w1266, w1267, w1265) -> (w1261:dbl)
      n713 = Divide(x=2.0, y=9.0) -> (x/y=w1260:dbl)
      n714 = Power Of X(1:-1.0 ("x"), 2:w1225) -> (0:w1259:dbl)
      n715 = for {
        tunnel: w1261 -> [w1332]
        tunnel: w1238 -> [w1331] mode=indexing
        tunnel: w1260 -> [w1330]
        tunnel: w1259 -> [w1329]
        tunnel: [w1305] -> w1258 mode=indexing
        tunnel: [w1304] -> w1257 mode=indexing
        tunnel: [w1303] -> w1256 mode=indexing
        tunnel: [w1302] -> w1255 mode=indexing
        tunnel: [w1301] -> w1254 mode=indexing
        tunnel: [w1300] -> w1253 mode=indexing
        tunnel: [w1299] -> w1252 mode=indexing
        w1323 = 2.5 ("y")
        w1324 = 1.5 ("y")
        w1325 = 0.5 ("y")
        w1326 = -0.5 ("y")
        w1327 = -1.5 ("y")
        w1328 = -2.5 ("y")
        n716 = Subtract(x=w1331, y=w1332) -> (x-y=w1298:dbl)
        n717 = Multiply(x=w1298, y=w1329) -> (x*y=w1297:dbl)
        n718 = Add(x=w1330, y=w1297) -> (x+y=w1296:dbl)
        n719 = Less Or Equal?(x=w1296, y=w1324) -> (x <= y?=w1317:bool)
        n720 = Less Or Equal?(x=w1296, y=w1325) -> (x <= y?=w1315:bool)
        n721 = Greater?(x=w1296, y=w1325) -> (0:w1318:bool)
        n722 = Greater?(x=w1296, y=w1323) -> (0:w1311:bool)
        n723 = Less Or Equal?(x=w1296, y=w1326) -> (x <= y?=w1313:bool)
        n724 = Greater?(x=w1296, y=w1326) -> (0:w1316:bool)
        n725 = Less Or Equal?(x=w1296, y=w1323) -> (x <= y?=w1319:bool)
        n726 = Less Or Equal?(x=w1296, y=w1327) -> (x <= y?=w1321:bool)
        n727 = Greater?(x=w1296, y=w1327) -> (0:w1314:bool)
        n728 = Greater?(x=w1296, y=w1324) -> (0:w1320:bool)
        n729 = Less Or Equal?(x=w1296, y=w1328) -> (x <= y?=w1312:bool)
        n730 = Greater?(x=w1296, y=w1328) -> (0:w1322:bool)
        n731 = And(x=w1320, y=w1319) -> (x .and. y?=w1306:bool)
        n732 = And(x=w1316, y=w1315) -> (x .and. y?=w1308:bool)
        n733 = And(x=w1318, y=w1317) -> (x .and. y?=w1307:bool)
        n734 = And(x=w1314, y=w1313) -> (x .and. y?=w1309:bool)
        n735 = And(x=w1322, y=w1321) -> (x .and. y?=w1310:bool)
        n736 = case shown="True" w1306 {
          tunnel: [0 1] -> w1300
          frame False {
          }
          frame True {
          }
        }
        n737 = case shown="True" w1311 {
          tunnel: [0 1] -> w1299
          frame False {
          }
          frame True {
          }
        }
        n738 = case shown="True" w1307 {
          tunnel: [0 1] -> w1301
          frame False {
          }
          frame True {
          }
        }
        n739 = case shown="True" w1308 {
          tunnel: [0 1] -> w1302
          frame False {
          }
          frame True {
          }
        }
        n740 = case shown="True" w1310 {
          tunnel: [0 1] -> w1304
          frame False {
          }
          frame True {
          }
        }
        n741 = case shown="True" w1309 {
          tunnel: [0 1] -> w1303
          frame False {
          }
          frame True {
          }
        }
        n742 = case shown="True" w1312 {
          tunnel: [0 1] -> w1305
          frame False {
          }
          frame True {
          }
        }
      }
      n743 = Add Array Elements(numeric array=w1253) -> (sum=w1246:i32)
      "v5 2" <- w1246
      n744 = Add Array Elements(numeric array=w1252) -> (sum=w1245:i32)
      "v6" <- w1245
      n745 = Add Array Elements(numeric array=w1257) -> (sum=w1250:i32)
      "v1 2" <- w1250
      n746 = Add Array Elements(numeric array=w1256) -> (sum=w1249:i32)
      "v2 2" <- w1249
      n747 = Add Array Elements(numeric array=w1254) -> (sum=w1247:i32)
      "v4 2" <- w1247
      n748 = Add Array Elements(numeric array=w1258) -> (sum=w1251:i32)
      "v0 2" <- w1251
      n749 = Add Array Elements(numeric array=w1255) -> (sum=w1248:i32)
      "v3 2" <- w1248
      n750 = Build Array(w1251, w1250, w1249, w1248, w1247, w1246, w1245) -> (w1244:i32[])
      n751 = for {
        tunnel: w1244 -> [w1293] mode=indexing
        tunnel: dbl[] [0.01047, 0.03125, 0.125, 0.5, 0.25, 0.0625, 0.020833] -> [w1294] mode=indexing
        tunnel: w1235 -> [w1295]
        tunnel: [w1289] -> w1243 mode=indexing
        n752 = Multiply(x=w1295, y=w1294) -> (x*y=w1290:dbl)
        n753 = Subtract(x=w1293, y=w1290) -> (x-y=w1292:dbl)
        n754 = Square(x=w1292) -> (x^2=w1291:dbl)
        n755 = Divide(x=w1291, y=w1290) -> (x/y=w1289:dbl)
      }
      n756 = Add Array Elements(numeric array=w1243) -> (sum=w1242:dbl)
      n757 = Divide(x=w1242, y=2.0) -> (x/y=w1240:dbl)
      n758 = call <vilib>:"Complementary Incomplete Gamma Function.vi"("a"=w1240, "x"=3.0) -> ("1 - g(x, a)"=w1229:dbl)  [unwired: 1 in]
      "?" <- w1229
      n759 = Greater Or Equal?(x=w1229, y=0.01) -> (x >= y?=w1231:bool)
      n760 = case shown="False" w1231 {
        tunnel: ["Failed" "Passed"] -> w1230
        frame False {
        }
        frame True {
        }
      }
      "?" <- w1230
    }
    frame #10 {
      n761 = Decimal String To Number(string=w1509) -> (number=w1510:i32[])  [unwired: 2 in, 1 out]
      n762 = Equal?(x="m", y=0) -> (x = y?=w1503:bool)
      n763 = Array Size(array=w1510) -> (size(s)=w1517:i32)
      n764 = case shown="True" w1503 {
        tunnel: [w1536 16] -> w1501
        tunnel: "m" -> [w1536 _]
        frame False {
        }
        frame True {
        }
      }
      n765 = for {
        N: w1501 -> [_]
        tunnel: [w1553] -> w1535 mode=indexing
        tunnel: w1510 -> [w1551]
        i -> [w1552]
        n766 = Add(x=1, y=w1552) -> (x+y=w1557:i32)
        n767 = Power Of 2(x=w1557) -> (2^x=w1556:dbl)
        n768 = for {
          N: w1556 -> [_]
          tunnel: [w1615] -> w1563 mode=indexing
          i -> [w1614]
          n769 = property on="Numeric 2" class="DigNum (strict)"() -> ("NumText.Text"=w1615:string)  [unwired: 2 in, 2 out]
          "Numeric 2" <- w1614
        }
        n770 = for {
          tunnel: w1563 -> [w1612] mode=indexing
          tunnel: [w1613] -> w1562 mode=indexing
          w1611 = "0" ("문자열")
          n771 = Concatenate Strings(w1611, w1611, w1611, w1611, w1611, w1611, w1611, w1611, w1611, w1611, w1611, w1611, w1611, w1611, w1611, w1611, w1611, w1611, w1611, w1611, w1611, w1612) -> (w1613:string)
        }
        n772 = for {
          tunnel: w1562 -> [w1609] mode=indexing
          tunnel: [w1608] -> w1561 mode=indexing
          tunnel: [w1606] -> w1560
          tunnel: w1557 -> [w1606]
          # "자리수"
          n773 = String Length(string=w1609) -> (length=w1610:i32)
          n774 = Subtract(x=w1610, y=w1606) -> (x-y=w1607:i32)
          n775 = String Subset(string=w1609, offset (0)=w1607, length (rest)=w1606) -> (substring=w1608:string)
        }
        n776 = for {
          tunnel: w1561 -> [w1601] mode=indexing
          tunnel: w1560 -> [w1600]
          tunnel: [w1599] -> w1559 mode=indexing
          n777 = for {
            N: w1600 -> [_]
            tunnel: w1601 -> [w1604]
            tunnel: [w1602] -> w1599 mode=indexing
            i -> [w1603]
            n778 = String Subset(string=w1604, offset (0)=w1603, length (rest)=1 ("길이(나머지)")) -> (substring=w1602:string)
          }
        }
        n779 = Decimal String To Number(string=w1559) -> (number=w1555:i32[][])  [unwired: 2 in, 1 out]
        n780 = for {
          N: 1 -> [_]
          tunnel: w1551 -> [w1570]
          tunnel: w1555 -> [w1567]
          tunnel: [w1566] -> w1553
          tunnel: w1552 -> [w1565]
          i -> [w1564]
          # "m=3,   m-1= 3-1= 2 bit 추가"
          n781 = Array Size(array=w1570) -> (size(s)=w1572:i32)
          n782 = Delete From Array(array=w1570, length=w1565, index=0 ("인덱스")) -> (deleted portion=w1573:i32[])  [unwired: 1 out]
          n783 = Add(x=1, y=w1565) -> (x+y=w1568:i32)
          n784 = Insert Into Array(array=w1570, index=w1572, new element=w1573) -> (w1571:i32[])
          n785 = Array Size(array=w1571) -> (size(s)=w1574:i32)
          n786 = for {
            tunnel: w1571 -> [w1581]
            tunnel: w1567 -> [w1580] mode=indexing
            tunnel: w1574 -> [w1579]
            tunnel: [w1578] -> w1566 mode=indexing
            tunnel: w1568 -> [w1577]
            n787 = for {
              N: w1579 -> [_]
              tunnel: w1581 -> [w1594]
              tunnel: w1580 -> [w1588]
              shift-right: [w1591] -> w1578
              shift-left: 0.0 -> [w1590]
              tunnel: w1577 -> [w1582]
              i -> [w1593]
              n788 = Array Subset(array=w1594, index=w1593, length=w1582) -> (w1589:i32[])
              n789 = Equal?(x=w1588, y=w1589) -> (x = y?=w1592:bool[])
              n790 = Array Size(array=w1588) -> (size(s)=w1586:i32)
              n791 = Array Size(array=w1589) -> (size(s)=w1587:i32)
              n792 = Equal?(x=w1586, y=w1587) -> (x = y?=w1585:bool)
              n793 = And Array Elements(Boolean array=w1592) -> (logical AND=w1584:bool)
              n794 = And(x=w1584, y=w1585) -> (x .and. y?=w1583:bool)
              n795 = case shown="False" w1583 {
                tunnel: [w1595 w1597] -> w1591
                tunnel: w1590 -> [w1595 w1596]
                frame False {
                }
                frame True {
                  n796 = Add(x=w1596, y=1.0) -> (x+y=w1597:dbl)
                }
              }
            }
          }
          "안에" <- w1564
        }
        "전체" <- w1552
      }
      n797 = for {
        tunnel: w1535 -> [w1546] mode=indexing
        tunnel: w1517 -> [w1547]
        tunnel: [w1540] -> w1534 mode=indexing
        i -> [w1543]
        n798 = Square(x=w1546) -> (x^2=w1545:dbl[])
        n799 = Add Array Elements(numeric array=w1545) -> (sum=w1544:dbl)
        n800 = Add(x=1, y=w1543) -> (x+y=w1541:i32)
        n801 = Power Of 2(x=w1541) -> (2^x=w1550:dbl)
        n802 = Divide(x=w1550, y=w1547) -> (x/y=w1549:dbl)
        n803 = Multiply(x=w1544, y=w1549) -> (x*y=w1548:dbl)
        n804 = Subtract(x=w1548, y=w1547) -> (x-y=w1540:dbl)
      }
      n805 = Reverse 1D Array(array=w1534) -> (reversed array=w1531:dbl[])
      n806 = Index Array(array=w1531, index=2) -> (element=w1527:dbl)
      n807 = Index Array(array=w1531, index=1) -> (element=w1529:dbl)
      n808 = Index Array(array=w1531, index=0) -> (element=w1525:dbl)
      n809 = Multiply(x=w1529, y=-2.0) -> (x*y=w1526:dbl)
      n810 = Subtract(x=w1525, y=w1529) -> (x-y=w1516:dbl)
      "델타 프사이" <- w1516
      n811 = Subtract(x=w1501, y=3) -> (x-y=w1521:i32)
      n812 = Subtract(x=w1501, y=2) -> (x-y=w1522:i32)
      n813 = Compound Arithmetic op=ADD(w1525, w1526, w1527) -> (w1512:dbl)
      "델타^2 프사이" <- w1512
      n814 = Power Of 2(x=w1522) -> (2^x=w1520:dbl)
      "2^(m-2)" <- w1520
      n815 = Power Of 2(x=w1521) -> (2^x=w1519:dbl)
      "2^(m-3)" <- w1519
      n816 = Divide(x=w1516, y=2.0) -> (x/y=w1514:dbl)
      n817 = Divide(x=w1512, y=2.0) -> (x/y=w1511:dbl)
      n818 = call <vilib>:"Complementary Incomplete Gamma Function.vi"("a"=w1514, "x"=w1520) -> ("1 - g(x, a)"=w1505:dbl)  [unwired: 1 in]
      "?" <- w1505
      n819 = call <vilib>:"Complementary Incomplete Gamma Function.vi"("a"=w1511, "x"=w1519) -> ("1 - g(x, a)"=→"p-value2":dbl)  [unwired: 1 in]
      n820 = Greater Or Equal?(x=w1505, y=0.01) -> (x >= y?=w1507:bool)
      n821 = case shown="False" w1507 {
        tunnel: ["Failed" "Passed"] -> w1506
        frame False {
        }
        frame True {
        }
      }
      "?" <- w1506
    }
    frame #11 {
      n822 = Decimal String To Number(string=w1620) -> (number=w1622:i32[])  [unwired: 2 in, 1 out]
      n823 = Array Size(array=w1622) -> (size(s)=w1621:i32)
      n824 = for {
        N: 2 -> [_]
        tunnel: [w1672] -> w1640 mode=indexing
        tunnel: w1622 -> [w1671]
        tunnel: [w1657] -> w1628
        i -> [w1662]
        n825 = Equal?(x="m 2", y=0) -> (x = y?=w1659:bool)
        n826 = case shown="False" w1659 {
          tunnel: [w1673 10] -> w1657
          tunnel: "m 2" -> [w1673 _]
          frame False {
          }
          frame True {
          }
        }
        n827 = Add(x=w1657, y=w1662) -> (x+y=w1661:i32)
        n828 = Power Of 2(x=w1661) -> (2^x=w1665:dbl)
        n829 = for {
          N: w1665 -> [_]
          tunnel: [w1724] -> w1670 mode=indexing
          i -> [w1723]
          n830 = property on="Numeric 3" class="DigNum (strict)"() -> ("NumText.Text"=w1724:string)  [unwired: 2 in, 2 out]
          "Numeric 3" <- w1723
        }
        n831 = for {
          tunnel: w1670 -> [w1721] mode=indexing
          tunnel: [w1722] -> w1669 mode=indexing
          w1720 = "0" ("문자열")
          n832 = Concatenate Strings(w1720, w1720, w1720, w1720, w1720, w1720, w1720, w1720, w1720, w1720, w1720, w1720, w1720, w1720, w1720, w1720, w1720, w1720, w1720, w1720, w1720, w1721) -> (w1722:string)
        }
        n833 = for {
          tunnel: w1669 -> [w1718] mode=indexing
          tunnel: [w1717] -> w1668 mode=indexing
          tunnel: [w1715] -> w1667
          tunnel: w1661 -> [w1715]
          # "자리수"
          n834 = String Length(string=w1718) -> (length=w1719:i32)
          n835 = Subtract(x=w1719, y=w1715) -> (x-y=w1716:i32)
          n836 = String Subset(string=w1718, offset (0)=w1716, length (rest)=w1715) -> (substring=w1717:string)
        }
        n837 = for {
          tunnel: w1668 -> [w1710] mode=indexing
          tunnel: w1667 -> [w1709]
          tunnel: [w1708] -> w1666 mode=indexing
          n838 = for {
            N: w1709 -> [_]
            tunnel: w1710 -> [w1713]
            tunnel: [w1711] -> w1708 mode=indexing
            i -> [w1712]
            n839 = String Subset(string=w1713, offset (0)=w1712, length (rest)=1 ("길이(나머지)")) -> (substring=w1711:string)
          }
        }
        n840 = Decimal String To Number(string=w1666) -> (number=w1664:i32[][])  [unwired: 2 in, 1 out]
        n841 = for {
          N: 1 -> [_]
          tunnel: w1671 -> [w1679]
          tunnel: w1664 -> [w1678]
          tunnel: [w1677] -> w1672
          tunnel: w1661 -> [w1675]
          # "m=3,   m-1= 3-1= 2 bit 추가"
          n842 = Decrement(x=w1675) -> (x-1=w1676:i32)
          n843 = Array Size(array=w1679) -> (size(s)=w1681:i32)
          n844 = Delete From Array(array=w1679, length=w1676, index=0 ("인덱스")) -> (deleted portion=w1682:i32[])  [unwired: 1 out]
          n845 = Insert Into Array(array=w1679, index=w1681, new element=w1682) -> (w1680:i32[])
          n846 = Array Size(array=w1680) -> (size(s)=w1683:i32)
          n847 = for {
            tunnel: w1680 -> [w1690]
            tunnel: w1678 -> [w1689] mode=indexing
            tunnel: w1683 -> [w1688]
            tunnel: [w1687] -> w1677 mode=indexing
            tunnel: w1675 -> [w1686]
            n848 = for {
              N: w1688 -> [_]
              tunnel: w1690 -> [w1703]
              tunnel: w1689 -> [w1697]
              shift-right: [w1700] -> w1687
              shift-left: 0.0 -> [w1699]
              tunnel: w1686 -> [w1691]
              i -> [w1702]
              n849 = Array Subset(array=w1703, index=w1702, length=w1691) -> (w1698:i32[])
              n850 = Equal?(x=w1697, y=w1698) -> (x = y?=w1701:bool[])
              n851 = Array Size(array=w1697) -> (size(s)=w1695:i32)
              n852 = Array Size(array=w1698) -> (size(s)=w1696:i32)
              n853 = Equal?(x=w1695, y=w1696) -> (x = y?=w1694:bool)
              n854 = And Array Elements(Boolean array=w1701) -> (logical AND=w1693:bool)
              n855 = And(x=w1693, y=w1694) -> (x .and. y?=w1692:bool)
              n856 = case shown="False" w1692 {
                tunnel: [w1704 w1706] -> w1700
                tunnel: w1699 -> [w1704 w1705]
                frame False {
                }
                frame True {
                  n857 = Add(x=w1705, y=1.0) -> (x+y=w1706:dbl)
                }
              }
            }
          }
        }
      }
      n858 = for {
        tunnel: w1640 -> [w1649] mode=indexing
        tunnel: w1621 -> [w1650]
        tunnel: [w1648] -> w1639 mode=indexing
        n859 = Divide(x=w1649, y=w1650) -> (x/y=w1646:dbl[])
        n860 = for {
          tunnel: w1646 -> [w1652] mode=indexing
          tunnel: [w1651] -> w1645 mode=indexing
          n861 = Equal?(x=w1652, y=0.0) -> (x = y?=w1653:bool)
          n862 = case shown="True" w1653 {
            tunnel: [w1655 1.0 ("y")] -> w1651
            tunnel: w1652 -> [w1655 _]
            frame False {
            }
            frame True {
            }
          }
        }
        n863 = Natural Logarithm(1:w1645) -> (0:w1644:dbl[])
        n864 = Multiply(x=w1644, y=w1646) -> (x*y=w1647:dbl[])
        n865 = Add Array Elements(numeric array=w1647) -> (sum=w1648:dbl)
      }
      n866 = Index Array(array=w1639, index=0) -> (element=w1636:dbl)
      n867 = Index Array(array=w1639, index=1) -> (element=w1635:dbl)
      n868 = Subtract(x=w1636, y=w1635) -> (x-y=w1632:dbl)
      "ApEn(m)" <- w1632
      n869 = Natural Logarithm(1:2.0 ("x")) -> (0:w1633:dbl)
      n870 = Subtract(x=w1633, y=w1632) -> (x-y=w1630:dbl)
      n871 = Multiply(x=w1621, y=2) -> (x*y=w1629:i32)
      n872 = Multiply(x=w1630, y=w1629) -> (x*y=w1625:dbl)
      "X^2 5" <- w1625
      n873 = Decrement(x=w1628) -> (x-1=w1627:i32)
      n874 = Divide(x=w1625, y=2.0) -> (x/y=w1623:dbl)
      n875 = Power Of 2(x=w1627) -> (2^x=w1626:dbl)
      n876 = call <vilib>:"Complementary Incomplete Gamma Function.vi"("a"=w1623, "x"=w1626) -> ("1 - g(x, a)"=w1616:dbl)  [unwired: 1 in]
      "?" <- w1616
      n877 = Greater Or Equal?(x=w1616, y=0.01) -> (x >= y?=w1618:bool)
      n878 = case shown="False" w1618 {
        tunnel: ["Failed" "Passed"] -> w1617
        frame False {
        }
        frame True {
        }
      }
      "?" <- w1617
    }
    frame #12 {
      n879 = Decimal String To Number(string=w1729) -> (number=w1730:i32[])  [unwired: 2 in, 1 out]
      n880 = Array Size(array=w1730) -> (size(s)=w1742:i32)
      n881 = Multiply(x=w1730, y=2) -> (x*y=w1750:i32[])
      n882 = Subtract(x=w1750, y=1) -> (x-y=w1746:i32[])
      n883 = Reverse 1D Array(array=w1746) -> (reversed array=w1745:i32[])
      n884 = for {
        tunnel: w1745 -> [w1852] mode=indexing
        shift-right: [w1851] -> _
        shift-left: 0 -> [w1853]
        tunnel: [w1851] -> w1743 mode=indexing
        n885 = Add(x=w1853, y=w1852) -> (x+y=w1851:i32)
      }
      n886 = for {
        tunnel: w1746 -> [w1855] mode=indexing
        shift-right: [w1854] -> _
        shift-left: 0 -> [w1856]
        tunnel: [w1854] -> w1748 mode=indexing
        n887 = Add(x=w1856, y=w1855) -> (x+y=w1854:i32)
      }
      n888 = Add(x=0, y=w1742) -> (x+y=w1738:i32)
      n889 = Absolute Value(x=w1743) -> (abs(x)=w1744:i32[])
      n890 = Absolute Value(x=w1748) -> (abs(x)=w1747:i32[])
      n891 = Array Max & Min(array=w1744) -> (max value=w1736:i32)  [unwired: 3 out]
      "backward max value" <- w1736
      n892 = Array Max & Min(array=w1747) -> (max value=w1737:i32)  [unwired: 3 out]
      "forward max value" <- w1737
      n893 = Build Array(w1737, w1736) -> (w1735:i32[])
      n894 = for {
        tunnel: w1738 -> [w1767]
        tunnel: w1735 -> [w1758] mode=indexing
        tunnel: [w1757] -> w1733 mode=indexing
        n895 = Negate(x=w1767) -> (-x=w1787:i32)
        n896 = Negate(x=w1767) -> (-x=w1794:i32)
        n897 = Square Root(x=w1767) -> (sqrt(x)=w1759:dbl)
        n898 = Divide(x=w1767, y=w1758) -> (x/y=w1766:dbl)
        n899 = Divide(x=w1787, y=w1758) -> (x/y=w1764:dbl)
        n900 = Divide(x=w1794, y=w1758) -> (x/y=w1793:dbl)
        n901 = Divide(x=w1767, y=w1758) -> (x/y=w1790:dbl)
        n902 = Decrement(x=w1766) -> (x-1=w1765:dbl)
        n903 = Subtract(x=w1764, y=3.0) -> (x-y=w1762:dbl)
        n904 = Decrement(x=w1790) -> (x-1=w1788:dbl)
        n905 = Increment(x=w1793) -> (x+1=w1792:dbl)
        n906 = Divide(x=w1762, y=4.0) -> (x/y=w1776:dbl)
        n907 = Divide(x=w1792, y=4.0) -> (x/y=w1769:dbl)
        n908 = Divide(x=w1765, y=4.0) -> (x/y=w1777:dbl)
        n909 = Divide(x=w1788, y=4.0) -> (x/y=w1768:dbl)
        n910 = while {
          tunnel: w1776 -> [w1825]
          tunnel: w1777 -> [w1823]
          tunnel: [w1821] -> w1780 mode=indexing
          i -> [w1824]
          stop <- w1822 stop-if-true
          n911 = Add(x=w1824, y=w1825) -> (x+y=w1820:dbl)
          n912 = Less?(x=w1823, y=w1820) -> (x < y?=w1822:bool)
          n913 = Round Toward +Infinity(x=w1820) -> (ceil(x): smallest int >= x=w1821:dbl)
        }
        n914 = while {
          tunnel: w1769 -> [w1831]
          tunnel: w1768 -> [w1829]
          tunnel: [w1826] -> w1783 mode=indexing
          i -> [w1830]
          stop <- w1828 stop-if-true
          n915 = Add(x=w1830, y=w1831) -> (x+y=w1827:dbl)
          n916 = Less?(x=w1829, y=w1827) -> (x < y?=w1828:bool)
          n917 = Round Toward +Infinity(x=w1827) -> (ceil(x): smallest int >= x=w1826:dbl)
        }
        n918 = Array Size(array=w1783) -> (size(s)=w1782:i32)
        n919 = Decrement(x=w1782) -> (x-1=w1781:i32)
        n920 = Delete From Array(array=w1783, index=w1781) -> (array with subset deleted=w1755:dbl[])  [unwired: 1 in, 1 out]
        n921 = Array Size(array=w1780) -> (size(s)=w1779:i32)
        n922 = Decrement(x=w1779) -> (x-1=w1778:i32)
        n923 = Delete From Array(array=w1780, index=w1778) -> (array with subset deleted=w1775:dbl[])  [unwired: 1 in, 1 out]
        n924 = for {
          tunnel: [w1803] -> w1772 mode=indexing
          tunnel: w1775 -> [w1800] mode=indexing
          tunnel: w1759 -> [w1797]
          tunnel: w1758 -> [w1802]
          tunnel: [w1798] -> w1771 mode=indexing
          w1799 = 4.0 ("x")
          n925 = Multiply(x=w1799, y=w1800) -> (x*y=w1804:dbl)
          n926 = Multiply(x=w1800, y=w1799) -> (x*y=w1807:dbl)
          n927 = Increment(x=w1804) -> (x+1=w1801:dbl)
          n928 = Add(x=w1807, y=3.0) -> (x+y=w1805:dbl)
          n929 = Multiply(x=w1805, y=w1802) -> (x*y=w1796:dbl)
          n930 = Multiply(x=w1802, y=w1801) -> (x*y=w1795:dbl)
          n931 = Divide(x=w1796, y=w1797) -> (x/y=w1803:dbl)
          n932 = Divide(x=w1795, y=w1797) -> (x/y=w1798:dbl)
        }
        n933 = for {
          tunnel: [w1809] -> w1773 mode=indexing
          tunnel: [w1808] -> w1774 mode=indexing
          tunnel: w1759 -> [w1812]
          tunnel: w1758 -> [w1813]
          tunnel: w1755 -> [w1811] mode=indexing
          w1810 = 4.0 ("x")
          n934 = Multiply(x=w1811, y=w1810) -> (x*y=w1819:dbl)
          n935 = Multiply(x=w1810, y=w1811) -> (x*y=w1817:dbl)
          n936 = Decrement(x=w1817) -> (x-1=w1816:dbl)
          n937 = Increment(x=w1819) -> (x+1=w1815:dbl)
          n938 = Multiply(x=w1816, y=w1813) -> (x*y=w1818:dbl)
          n939 = Multiply(x=w1815, y=w1813) -> (x*y=w1814:dbl)
          n940 = Divide(x=w1814, y=w1812) -> (x/y=w1808:dbl)
          n941 = Divide(x=w1818, y=w1812) -> (x/y=w1809:dbl)
        }
        n942 = Build Array(w1774, w1773, w1772, w1771) -> (w1756:dbl[][])
        n943 = for {
          tunnel: w1756 -> [w1846] mode=indexing
          tunnel: [w1845] -> w1770 mode=indexing
          n944 = for {
            tunnel: w1846 -> [w1848] mode=indexing
            tunnel: [w1847] -> w1845 mode=indexing
            n945 = call-poly <vilib>:"Continuous CDF.vi"("std"=1.0, "mean"=0.0, "x"=w1848) -> ("cdf(x)"=w1847:dbl)  [unwired: 7 in, 1 out]
          }
        }
        n946 = Transpose Matrix(1:w1770) -> (0:w1754:dbl[][])
        n947 = for {
          tunnel: w1754 -> [w1838] mode=indexing
          tunnel: [w1835] -> w1784 mode=indexing
          n948 = Index Array(array=w1838, index=0) -> (element=w1842:dbl)
          n949 = Index Array(array=w1838, index=1) -> (element=w1841:dbl)
          n950 = Index Array(array=w1838, index=2) -> (element=w1837:dbl)
          n951 = Index Array(array=w1838, index=3) -> (element=w1836:dbl)
          n952 = Subtract(x=w1842, y=w1841) -> (x-y=w1833:dbl)
          n953 = Subtract(x=w1837, y=w1836) -> (x-y=w1834:dbl)
          n954 = Negate(x=w1833) -> (-x=w1832:dbl)
          n955 = Add(x=w1832, y=w1834) -> (x+y=w1835:dbl)
        }
        n956 = Add Array Elements(numeric array=w1784) -> (sum=w1760:dbl)
        n957 = Add(x=1.0, y=w1760) -> (x+y=w1757:dbl)
      }
      n958 = Index Array(array=w1733, index=0) -> (element=w1725:dbl)
      "?" <- w1725
      "Forward P-value" <- w1725
      n959 = Index Array(array=w1733, index=1) -> (element=→"backward P-value":dbl)
      n960 = Greater Or Equal?(x=w1725, y=0.01) -> (x >= y?=w1727:bool)
      n961 = case shown="False" w1727 {
        tunnel: ["Failed" "Passed"] -> w1726
        frame False {
        }
        frame True {
        }
      }
      "?" <- w1726
    }
    frame #13 {
      w1874 = i32[] [4, 3, 2, 1, 1, 2, 3, 4]
      (unwired) dbl[][] [[0.875, 0.0156, 0.0137, 0.012, 0.0105, 0.0733], [0.8333, 0.0278, 0.0231, 0.0193, 0.0161, 0.0804], [0.75, 0.0625, 0.0469, 0.0352, 0.0264, 0.0791], [0.5, 0.25, 0.125, 0.0625, 0.0312, 0.0312], [0.5, 0.25, 0.125, 0.0625, 0.0312, 0.0312], [0.75, 0.0625, 0.0469, 0.0352, 0.0264, 0.0791], [0.8333, 0.0278, 0.0231, 0.0193, 0.0161, 0.0804], [0.875, 0.0156, 0.0137, 0.012, 0.0105, 0.0733]] ("y")
      # "파이 0 4개"
      # "s"
      # "x"
      n962 = Decimal String To Number(string=w1863) -> (number=w1886:i32[])  [unwired: 2 in, 1 out]
      n963 = Multiply(x=w1886, y=2) -> (x*y=w1904:i32[])
      n964 = Subtract(x=w1904, y=1) -> (x-y=w1902:i32[])
      n965 = for {
        tunnel: w1902 -> [w1986] mode=indexing
        shift-right: [w1985] -> _
        shift-left: 0 -> [w1987]
        tunnel: [w1985] -> w1898 mode=indexing
        n966 = Add(x=w1987, y=w1986) -> (x+y=w1985:i32)
      }
      n967 = Array Size(array=w1898) -> (size(s)=w1899:i32)
      n968 = Insert Into Array(array=w1898, index=w1899, new element=0 ("new element/subarray")) -> (w1897:i32[])
      n969 = while {
        shift-right: [w1977] -> _
        shift-left: w1897 -> [w1976]
        tunnel: [w1967] -> w1893 mode=indexing
        tunnel: [w1968] -> w1890
        tunnel: [w1967] -> _ mode=indexing
        i -> [w1968]
        stop <- w1971 stop-if-true
        w1974 = 0 ("index")
        n970 = call "Search Unsorted 1D Array.vim"("element"=0.0, "unsorted 1D array"=w1976) -> ("index of element"=w1973:i32)  [unwired: 9 in]
        n971 = Equal?(x=w1973, y=-1) -> (x = y?=w1971:bool)
        n972 = Increment(x=w1973) -> (x+1=w1978:i32)
        n973 = Split 1D Array(array=w1976, index=w1978) -> (first subarray=w1975:i32[], second subarray=w1977:i32[])
        n974 = Insert Into Array(array=w1975, index=w1974, new element=w1974) -> (w1970:i32[])
        n975 = for {
          tunnel: w1970 -> [w1984]
          tunnel: i32[] [-4, -3, -2, -1, 1, 2, 3, 4] -> [w1983] mode=indexing
          tunnel: [w1980] -> w1967 mode=indexing
          n976 = Equal?(x=w1983, y=w1984) -> (x = y?=w1982:bool[])
          n977 = Boolean To (0,1)(Boolean=w1982) -> (0, 1=w1981:i16[])
          n978 = Add Array Elements(numeric array=w1981) -> (sum=w1980:i16)
        }
        "J" <- w1968
      }
      n979 = Array Size(array=w1893) -> (size(s)=w1896:i32[])
      n980 = Index Array(array=w1896) -> (element=w1895:i32)  [unwired: 1 in]
      n981 = Decrement(x=w1895) -> (x-1=w1894:i32)
      n982 = Delete From Array(array=w1893, index (row)=w1894) -> (array with subset deleted=w1892:i16[][])  [unwired: 2 in, 1 out]
      n983 = Transpose 2D Array(2D array=w1892) -> (transposed array=w1891:i16[][])
      n984 = for {
        tunnel: w1891 -> [w1942] mode=indexing
        tunnel: w1890 -> [w1945]
        tunnel: [w1943] -> w1885 mode=indexing
        n985 = for {
          tunnel: w1942 -> [w1951]
          tunnel: i32[] [5] -> [w1949] mode=indexing
          tunnel: [w1947] -> w1938
          n986 = Greater Or Equal?(x=w1951, y=w1949) -> (x >= y?=w1950:bool[])
          n987 = Boolean To (0,1)(Boolean=w1950) -> (0, 1=w1948:i16[])
          n988 = Add Array Elements(numeric array=w1948) -> (sum=w1947:i16)
        }
        n989 = for {
          tunnel: w1942 -> [w1966]
          tunnel: i32[] [0, 1, 2, 3, 4, 5] -> [w1965] mode=indexing
          tunnel: [w1962] -> w1939 mode=indexing
          n990 = Equal?(x=w1966, y=w1965) -> (x = y?=w1964:bool[])
          n991 = Boolean To (0,1)(Boolean=w1964) -> (0, 1=w1963:i16[])
          n992 = Add Array Elements(numeric array=w1963) -> (sum=w1962:i16)
        }
        n993 = Replace Array Subset(array=w1939, new element=w1938, index=5) -> (w1936:i16[])
        n994 = Add Array Elements(numeric array=w1936) -> (sum=w1944:i16)
        n995 = Equal?(x=w1944, y=w1945) -> (x = y?=w1946:bool)
        n996 = case shown="True" w1946 {
          tunnel: w1936 -> [w1953 w1961]
          tunnel: w1945 -> [w1960 _]
          tunnel: w1944 -> [w1959 _]
          tunnel: [w1952 w1961] -> w1943
          frame False {
            n997 = Subtract(x=w1960, y=w1959) -> (x-y=w1956:i32)
            n998 = Index Array(array=w1953, index=5) -> (element=w1957:i16)
            n999 = Add(x=w1957, y=w1956) -> (x+y=w1954:i32)
            n1000 = Replace Array Subset(array=w1953, new element=w1954, index=5) -> (w1952:i16[])
          }
          frame True {
          }
        }
      }
      n1001 = for {
        tunnel: w1874 -> [w1915] mode=indexing
        tunnel: [w1908] -> w1867 mode=indexing
        n1002 = Multiply(x=2.0, y=w1915) -> (x*y=w1917:dbl)
        n1003 = Square(x=w1915) -> (x^2=w1914:i32)
        n1004 = Reciprocal(x=w1917) -> (1/x=w1916:dbl)
        n1005 = Multiply(x=w1914, y=4) -> (x*y=w1912:i32)
        n1006 = Reciprocal(x=w1912) -> (1/x=w1920:dbl)
        n1007 = Subtract(x=1.0, y=w1916) -> (x-y=w1911:dbl)
        n1008 = Power Of X(1:w1911, 2:i32[] [0, 1, 2, 3]) -> (0:w1909:dbl[])
        n1009 = Multiply(x=w1920, y=w1909) -> (x*y=w1908:dbl[])
      }
      n1010 = Multiply(x=2.0, y=w1874) -> (x*y=w1876:dbl[])
      n1011 = Multiply(x=2.0, y=w1874) -> (x*y=w1879:dbl[])
      n1012 = Reciprocal(x=w1876) -> (1/x=w1875:dbl[])
      n1013 = Reciprocal(x=w1879) -> (1/x=w1873:dbl[])
      n1014 = Subtract(x=1.0, y=w1875) -> (x-y=w1872:dbl[])
      n1015 = Power Of X(1:w1872, 2:4.0 ("x")) -> (0:w1870:dbl[])
      n1016 = Multiply(x=2.0, y=w1874) -> (x*y=w1882:dbl[])
      n1017 = Reciprocal(x=w1882) -> (1/x=w1881:dbl[])
      n1018 = Subtract(x=1.0, y=w1881) -> (x-y=w1869:dbl[])
      n1019 = Multiply(x=w1870, y=w1873) -> (x*y=w1868:dbl[])
      n1020 = Transpose 2D Array(2D array=w1867) -> (transposed array=w1866:dbl[][])
      n1021 = Build Array (concatenate)(w1869, w1866, w1868) -> (w1865:dbl[][])
      n1022 = Transpose 2D Array(2D array=w1865) -> (transposed array=w1864:dbl[][])
      n1023 = for {
        tunnel: w1885 -> [w1928] mode=indexing
        tunnel: w1890 -> [w1927]
        tunnel: [w1925] -> w1889 mode=indexing
        tunnel: w1864 -> [w1924] mode=indexing
        n1024 = for {
          tunnel: w1928 -> [w1935] mode=indexing
          tunnel: w1927 -> [w1934]
          tunnel: w1924 -> [w1930] mode=indexing
          tunnel: [w1929] -> w1926 mode=indexing
          n1025 = Multiply(x=w1934, y=w1930) -> (x*y=w1931:dbl)
          n1026 = Subtract(x=w1935, y=w1931) -> (x-y=w1933:dbl)
          n1027 = Square(x=w1933) -> (x^2=w1932:dbl)
          n1028 = Divide(x=w1932, y=w1931) -> (x/y=w1929:dbl)
        }
        n1029 = Add Array Elements(numeric array=w1926) -> (sum=w1925:dbl)
      }
      "X^2 6" <- w1889
      n1030 = Divide(x=w1889, y=2.0 ("x")) -> (x/y=w1887:dbl[])
      n1031 = for {
        tunnel: w1887 -> [w1922] mode=indexing
        tunnel: [w1921] -> w1862 mode=indexing
        n1032 = call <vilib>:"Complementary Incomplete Gamma Function.vi"("a"=w1922, "x"=2.5) -> ("1 - g(x, a)"=w1921:dbl)  [unwired: 1 in]
      }
      "P- VALUE" <- w1862
      n1033 = Index Array(array=w1862, index=4) -> (element=w1857:dbl)
      "?" <- w1857
      n1034 = Greater Or Equal?(x=w1857, y=0.01) -> (x >= y?=w1859:bool)
      n1035 = case shown="False" w1859 {
        tunnel: ["Failed" "Passed"] -> w1858
        frame False {
        }
        frame True {
        }
      }
      "?" <- w1858
    }
    frame #14 {
      n1036 = Decimal String To Number(string=w1994) -> (number=w1995:i32[])  [unwired: 2 in, 1 out]
      n1037 = Multiply(x=w1995, y=2) -> (x*y=w2012:i32[])
      n1038 = Subtract(x=w2012, y=1) -> (x-y=w2010:i32[])
      n1039 = for {
        tunnel: w2010 -> [w2052] mode=indexing
        shift-right: [w2051] -> _
        shift-left: 0 -> [w2053]
        tunnel: [w2051] -> w2006 mode=indexing
        n1040 = Add(x=w2053, y=w2052) -> (x+y=w2051:i32)
      }
      n1041 = Array Size(array=w2006) -> (size(s)=w2007:i32)
      n1042 = Insert Into Array(array=w2006, index=w2007, new element=0 ("new element/subarray")) -> (w2005:i32[])
      n1043 = while {
        shift-right: [w2043] -> _
        shift-left: w2005 -> [w2042]
        tunnel: [w2034] -> w2001 mode=indexing
        tunnel: [w2033] -> w1998
        i -> [w2033]
        stop <- w2037 stop-if-true
        w2040 = 0 ("index")
        n1044 = call "Search Unsorted 1D Array.vim"("element"=0.0, "unsorted 1D array"=w2042) -> ("index of element"=w2039:i32)  [unwired: 9 in]
        n1045 = Equal?(x=w2039, y=-1) -> (x = y?=w2037:bool)
        n1046 = Increment(x=w2039) -> (x+1=w2044:i32)
        n1047 = Split 1D Array(array=w2042, index=w2044) -> (first subarray=w2041:i32[], second subarray=w2043:i32[])
        n1048 = Insert Into Array(array=w2041, index=w2040, new element=w2040) -> (w2036:i32[])
        n1049 = for {
          tunnel: w2036 -> [w2050]
          tunnel: i32[] [-9, -8, -7, -6, -5, -4, -3, -2, -1, 1, 2, 3, 4, 5, 6, 7, 8, 9] -> [w2049] mode=indexing
          tunnel: [w2046] -> w2034 mode=indexing
          n1050 = Equal?(x=w2049, y=w2050) -> (x = y?=w2048:bool[])
          n1051 = Boolean To (0,1)(Boolean=w2048) -> (0, 1=w2047:i16[])
          n1052 = Add Array Elements(numeric array=w2047) -> (sum=w2046:i16)
        }
        "J" <- w2033
      }
      n1053 = Array Size(array=w2001) -> (size(s)=w2004:i32[])
      n1054 = Index Array(array=w2004) -> (element=w2003:i32)  [unwired: 1 in]
      n1055 = Decrement(x=w2003) -> (x-1=w2002:i32)
      n1056 = Delete From Array(array=w2001, index (row)=w2002) -> (array with subset deleted=w2000:i16[][])  [unwired: 2 in, 1 out]
      n1057 = Transpose 2D Array(2D array=w2000) -> (transposed array=w1999:i16[][])
      n1058 = for {
        tunnel: w1999 -> [w2032] mode=indexing
        tunnel: w1998 -> [w2021]
        tunnel: i32[] [-9, -8, -7, -6, -5, -4, -3, -2, -1, 1, 2, 3, 4, 5, 6, 7, 8, 9] -> [w2027] mode=indexing
        tunnel: [w2018] -> w1996 mode=indexing
        w2023 = 2.0 ("y")
        n1059 = Absolute Value(x=w2027) -> (abs(x)=w2026:i32)
        n1060 = Add Array Elements(numeric array=w2032) -> (sum=w2031:i16)
        n1061 = Subtract(x=w2031, y=w2021) -> (x-y=w2030:i32)
        n1062 = Absolute Value(x=w2030) -> (abs(x)=w2029:i32)
        n1063 = Multiply(x=w2026, y=4.0) -> (x*y=w2025:dbl)
        n1064 = Subtract(x=w2025, y=w2023) -> (x-y=w2024:dbl)
        n1065 = Multiply(x=w2024, y=w2023) -> (x*y=w2022:dbl)
        n1066 = Multiply(x=w2022, y=w2021) -> (x*y=w2020:dbl)
        n1067 = Square Root(x=w2020) -> (sqrt(x)=w2019:dbl)
        n1068 = Divide(x=w2029, y=w2019) -> (x/y=w2018:dbl)
      }
      n1069 = for {
        tunnel: w1996 -> [w2017] mode=indexing
        tunnel: [w2016] -> w1992 mode=indexing
        n1070 = call <vilib>:"Error Function Complement.vi"("x"=w2017) -> ("1 - erf(x)"=w2016:dbl)  [unwired: 2 in]
      }
      "P-VALUE" <- w1992
      n1071 = Index Array(array=w1992, index=8) -> (element=w1990:dbl)
      "?" <- w1990
      n1072 = Greater Or Equal?(x=w1990, y=0.01) -> (x >= y?=w1989:bool)
      n1073 = case shown="False" w1989 {
        tunnel: ["Failed" "Passed"] -> w1988
        frame False {
        }
        frame True {
        }
      }
      "?" <- w1988
    }
  }
